vi "Constellation diagram wizard.vi"() -> ()   [LabVIEW 2010]
uses:
  <vilib>/Waveform/DTblOps.llb/DTbl Invert Digital.vi
  <vilib>/Waveform/DTblOps.llb/DTbl Digital Size.vi
  <vilib>/Waveform/DTblOps.llb/DTbl Digital to Binary U32.vi
panel:
  in  "Цвет подписей точек":u32(colorbox)=6618880
  in  "Перемешать соотношения":bool
  out "digital waveform":digitalwaveform(waveform)={"t0"=timestamp(0 s since 1904-01-01), "dt"=0.01, "Y"={"transitions"=[], "data"=[[1, 0, 0], [0, 0, 1], [1, 0, 1], [0, 1, 1], [0, 0, 0], [1, 0, 0], [0, 0, 1], [0, 0, 0], [1, 1, 0], [1, 0, 0], [0, 1, 0], [0, 1, 0], [0, 1, 0], [0, 1, 1], [0, 1, 1], [1, 1, 1], [1, 0, 1], [0, 1, 0], [1, 0, 1], [1, 0, 1], [0, 0, 1], [0, 1, 0], [0, 1, 1], [1, 0, 1], [1, 0, 0], [1, 1, 0], [1, 1, 1], [1, 0, 0], [1, 0, 1], [1, 0, 1], [0, 1, 0], [0, 1, 1], [1, 1, 1], [0, 1, 0], [1, 1, 0], [1, 0, 0], [1, 0, 0], [0, 0, 0], [1, 0, 1], [0, 1, 1], [0, 1, 1], [0, 0, 0], [1, 1, 1], [0, 0, 1], [0, 1, 1], [0, 0, 0], [0, 1, 1], [0, 1, 0], [1, 1, 1], [1, 1, 1], [1, 0, 0], [1, 1, 1], [1, 0, 0], [0, 1, 1], [1, 0, 1], [0, 1, 0], [1, 0, 0], [0, 0, 1], [1, 0, 0], [0, 1, 0], [0, 0, 0], [1, 0, 1], [1, 0, 0], [0, 1, 1], [0, 0, 1], [1, 1, 0], [0, 0, 1], [1, 0, 1], [0, 0, 1], [0, 0, 1], [1, 1, 1], [0, 1, 0], [1, 1, 0], [0, 0, 1], [0, 0, 0], [1, 1, 1], [0, 1, 1], [0, 0, 0], [0, 0, 0], [0, 0, 1], [0, 0, 1], [1, 0, 0], [0, 1, 1], [0, 1, 1], [1, 1, 0], [1, 0, 0], [1, 1, 0], [0, 0, 1], [1, 1, 0], [1, 1, 1], [0, 0, 1], [0, 0, 1], [1, 1, 0], [1, 0, 1], [0, 0, 0], [1, 1, 0], [0, 0, 0], [0, 0, 1], [1, 1, 0], [0, 1, 0]]}}
  out "Количество ПБ":ext=8.0
  out "Временная диаграмма каналов":digitalwaveform(graph)={"t0"=timestamp(0 s since 1904-01-01), "dt"=0.01, "Y"={"transitions"=[], "data"=[[1, 0, 0], [0, 0, 1], [1, 0, 1], [0, 1, 1], [0, 0, 0], [1, 0, 0], [0, 0, 1], [0, 0, 0], [1, 1, 0], [1, 0, 0], [0, 1, 0], [0, 1, 0], [0, 1, 0], [0, 1, 1], [0, 1, 1], [1, 1, 1], [1, 0, 1], [0, 1, 0], [1, 0, 1], [1, 0, 1], [0, 0, 1], [0, 1, 0], [0, 1, 1], [1, 0, 1], [1, 0, 0], [1, 1, 0], [1, 1, 1], [1, 0, 0], [1, 0, 1], [1, 0, 1], [0, 1, 0], [0, 1, 1], [1, 1, 1], [0, 1, 0], [1, 1, 0], [1, 0, 0], [1, 0, 0], [0, 0, 0], [1, 0, 1], [0, 1, 1], [0, 1, 1], [0, 0, 0], [1, 1, 1], [0, 0, 1], [0, 1, 1], [0, 0, 0], [0, 1, 1], [0, 1, 0], [1, 1, 1], [1, 1, 1], [1, 0, 0], [1, 1, 1], [1, 0, 0], [0, 1, 1], [1, 0, 1], [0, 1, 0], [1, 0, 0], [0, 0, 1], [1, 0, 0], [0, 1, 0], [0, 0, 0], [1, 0, 1], [1, 0, 0], [0, 1, 1], [0, 0, 1], [1, 1, 0], [0, 0, 1], [1, 0, 1], [0, 0, 1], [0, 0, 1], [1, 1, 1], [0, 1, 0], [1, 1, 0], [0, 0, 1], [0, 0, 0], [1, 1, 1], [0, 1, 1], [0, 0, 0], [0, 0, 0], [0, 0, 1], [0, 0, 1], [1, 0, 0], [0, 1, 1], [0, 1, 1], [1, 1, 0], [1, 0, 0], [1, 1, 0], [0, 0, 1], [1, 1, 0], [1, 1, 1], [0, 0, 1], [0, 0, 1], [1, 1, 0], [1, 0, 1], [0, 0, 0], [1, 1, 0], [0, 0, 0], [0, 0, 1], [1, 1, 0], [0, 1, 0]]}}
  out "Точки карты после разметки":cluster{"I":dbl, "Q":dbl, "ПБ":u32}[](array[cluster])=[{"I"=6.0, "Q"=0.0, "ПБ"=4}, {"I"=-4.0, "Q"=4.0, "ПБ"=1}, {"I"=-4.0, "Q"=-4.0, "ПБ"=5}, {"I"=-6.0, "Q"=0.0, "ПБ"=3}, {"I"=0.0, "Q"=6.0, "ПБ"=0}, {"I"=6.0, "Q"=0.0, "ПБ"=4}, {"I"=-4.0, "Q"=4.0, "ПБ"=1}, {"I"=0.0, "Q"=6.0, "ПБ"=0}, {"I"=4.0, "Q"=-4.0, "ПБ"=6}, {"I"=6.0, "Q"=0.0, "ПБ"=4}, {"I"=4.0, "Q"=4.0, "ПБ"=2}, {"I"=4.0, "Q"=4.0, "ПБ"=2}, {"I"=4.0, "Q"=4.0, "ПБ"=2}, {"I"=-6.0, "Q"=0.0, "ПБ"=3}, {"I"=-6.0, "Q"=0.0, "ПБ"=3}, {"I"=0.0, "Q"=-6.0, "ПБ"=7}, {"I"=-4.0, "Q"=-4.0, "ПБ"=5}, {"I"=4.0, "Q"=4.0, "ПБ"=2}, {"I"=-4.0, "Q"=-4.0, "ПБ"=5}, {"I"=-4.0, "Q"=-4.0, "ПБ"=5}, {"I"=-4.0, "Q"=4.0, "ПБ"=1}, {"I"=4.0, "Q"=4.0, "ПБ"=2}, {"I"=-6.0, "Q"=0.0, "ПБ"=3}, {"I"=-4.0, "Q"=-4.0, "ПБ"=5}, {"I"=6.0, "Q"=0.0, "ПБ"=4}, {"I"=4.0, "Q"=-4.0, "ПБ"=6}, {"I"=0.0, "Q"=-6.0, "ПБ"=7}, {"I"=6.0, "Q"=0.0, "ПБ"=4}, {"I"=-4.0, "Q"=-4.0, "ПБ"=5}, {"I"=-4.0, "Q"=-4.0, "ПБ"=5}, {"I"=4.0, "Q"=4.0, "ПБ"=2}, {"I"=-6.0, "Q"=0.0, "ПБ"=3}, {"I"=0.0, "Q"=-6.0, "ПБ"=7}, {"I"=4.0, "Q"=4.0, "ПБ"=2}, {"I"=4.0, "Q"=-4.0, "ПБ"=6}, {"I"=6.0, "Q"=0.0, "ПБ"=4}, {"I"=6.0, "Q"=0.0, "ПБ"=4}, {"I"=0.0, "Q"=6.0, "ПБ"=0}, {"I"=-4.0, "Q"=-4.0, "ПБ"=5}, {"I"=-6.0, "Q"=0.0, "ПБ"=3}, {"I"=-6.0, "Q"=0.0, "ПБ"=3}, {"I"=0.0, "Q"=6.0, "ПБ"=0}, {"I"=0.0, "Q"=-6.0, "ПБ"=7}, {"I"=-4.0, "Q"=4.0, "ПБ"=1}, {"I"=-6.0, "Q"=0.0, "ПБ"=3}, {"I"=0.0, "Q"=6.0, "ПБ"=0}, {"I"=-6.0, "Q"=0.0, "ПБ"=3}, {"I"=4.0, "Q"=4.0, "ПБ"=2}, {"I"=0.0, "Q"=-6.0, "ПБ"=7}, {"I"=0.0, "Q"=-6.0, "ПБ"=7}, {"I"=6.0, "Q"=0.0, "ПБ"=4}, {"I"=0.0, "Q"=-6.0, "ПБ"=7}, {"I"=6.0, "Q"=0.0, "ПБ"=4}, {"I"=-6.0, "Q"=0.0, "ПБ"=3}, {"I"=-4.0, "Q"=-4.0, "ПБ"=5}, {"I"=4.0, "Q"=4.0, "ПБ"=2}, {"I"=6.0, "Q"=0.0, "ПБ"=4}, {"I"=-4.0, "Q"=4.0, "ПБ"=1}, {"I"=6.0, "Q"=0.0, "ПБ"=4}, {"I"=4.0, "Q"=4.0, "ПБ"=2}, {"I"=0.0, "Q"=6.0, "ПБ"=0}, {"I"=-4.0, "Q"=-4.0, "ПБ"=5}, {"I"=6.0, "Q"=0.0, "ПБ"=4}, {"I"=-6.0, "Q"=0.0, "ПБ"=3}, {"I"=-4.0, "Q"=4.0, "ПБ"=1}, {"I"=4.0, "Q"=-4.0, "ПБ"=6}, {"I"=-4.0, "Q"=4.0, "ПБ"=1}, {"I"=-4.0, "Q"=-4.0, "ПБ"=5}, {"I"=-4.0, "Q"=4.0, "ПБ"=1}, {"I"=-4.0, "Q"=4.0, "ПБ"=1}, {"I"=0.0, "Q"=-6.0, "ПБ"=7}, {"I"=4.0, "Q"=4.0, "ПБ"=2}, {"I"=4.0, "Q"=-4.0, "ПБ"=6}, {"I"=-4.0, "Q"=4.0, "ПБ"=1}, {"I"=0.0, "Q"=6.0, "ПБ"=0}, {"I"=0.0, "Q"=-6.0, "ПБ"=7}, {"I"=-6.0, "Q"=0.0, "ПБ"=3}, {"I"=0.0, "Q"=6.0, "ПБ"=0}, {"I"=0.0, "Q"=6.0, "ПБ"=0}, {"I"=-4.0, "Q"=4.0, "ПБ"=1}, {"I"=-4.0, "Q"=4.0, "ПБ"=1}, {"I"=6.0, "Q"=0.0, "ПБ"=4}, {"I"=-6.0, "Q"=0.0, "ПБ"=3}, {"I"=-6.0, "Q"=0.0, "ПБ"=3}, {"I"=4.0, "Q"=-4.0, "ПБ"=6}, {"I"=6.0, "Q"=0.0, "ПБ"=4}, {"I"=4.0, "Q"=-4.0, "ПБ"=6}, {"I"=-4.0, "Q"=4.0, "ПБ"=1}, {"I"=4.0, "Q"=-4.0, "ПБ"=6}, {"I"=0.0, "Q"=-6.0, "ПБ"=7}, {"I"=-4.0, "Q"=4.0, "ПБ"=1}, {"I"=-4.0, "Q"=4.0, "ПБ"=1}, {"I"=4.0, "Q"=-4.0, "ПБ"=6}, {"I"=-4.0, "Q"=-4.0, "ПБ"=5}, {"I"=0.0, "Q"=6.0, "ПБ"=0}, {"I"=4.0, "Q"=-4.0, "ПБ"=6}, {"I"=0.0, "Q"=6.0, "ПБ"=0}, {"I"=-4.0, "Q"=4.0, "ПБ"=1}, {"I"=4.0, "Q"=-4.0, "ПБ"=6}, {"I"=4.0, "Q"=4.0, "ПБ"=2}] {"ПБ" items=["0", "1", "10", "11", "100", "101", "110", "111"]}
  in  "Все возможные точки карты":cluster{"I":dbl, "Q":dbl, "ПБ":u32}[](array[cluster])=[{"I"=0.0, "Q"=6.0, "ПБ"=0}, {"I"=-4.0, "Q"=4.0, "ПБ"=1}, {"I"=4.0, "Q"=4.0, "ПБ"=2}, {"I"=-6.0, "Q"=0.0, "ПБ"=3}, {"I"=6.0, "Q"=0.0, "ПБ"=4}, {"I"=-4.0, "Q"=-4.0, "ПБ"=5}, {"I"=4.0, "Q"=-4.0, "ПБ"=6}, {"I"=0.0, "Q"=-6.0, "ПБ"=7}] {"ПБ" items=["0", "1", "10", "11", "100", "101", "110", "111"]}
  in  "Соотношение точек с ПБ":u8(ring) items=["По возрастанию", "По убыванию", "Пользовательское"]
  in  "Стоп":bool
  in  "Интервалы и смещения":T1={"Q смещение"=0.0, "Q интервал"=2.0, "I смещение"=0.0, "I интервал"=2.0} {"I интервал" min=1.0 step=1.0; "Q интервал" min=1.0 step=1.0}
  out "Количество точек":i32=8
  in  "Добавлять точки при\nувеличении размера карты":bool=TRUE
  in  "Очистить полностью":bool
  in  "Заполнить полностью":bool
  in  "Точки карты (позиции)":bool[][](array[boolean])=[[FALSE, FALSE, FALSE, TRUE, FALSE, FALSE, FALSE], [FALSE, TRUE, FALSE, FALSE, FALSE, TRUE, FALSE], [FALSE, FALSE, FALSE, FALSE, FALSE, FALSE, FALSE], [TRUE, FALSE, FALSE, FALSE, FALSE, FALSE, TRUE], [FALSE, FALSE, FALSE, FALSE, FALSE, FALSE, FALSE], [FALSE, TRUE, FALSE, FALSE, FALSE, TRUE, FALSE], [FALSE, FALSE, FALSE, TRUE, FALSE, FALSE, FALSE]]
  in  "Размер карты (N*N)":i32(slide)=7 min=1 max=8 step=1 scale=0.0..8.0
  in  "Показать подписи точек на карте":bool=TRUE
  in  "Смещение подписей":cluster{"I":dbl, "Q":dbl}={"I"=0.0, "Q"=0.5}
  in  "Путь для загрузки карты":path=path "C:/Users/fl1ckje/Desktop/OFDM/map.xml"
  in  "Загрузить карту из файла":bool
  in  "Путь для сохранения карты":path=path "C:/Users/fl1ckje/Desktop/OFDM/map.xml"
  in  "Сохранить карту в файл":bool
  out "Карта":cluster{cluster{"I":dbl, "Q":dbl}[]}[](graph)=[{[{"I"=0.0, "Q"=6.0}, {"I"=-4.0, "Q"=4.0}, {"I"=4.0, "Q"=4.0}, {"I"=-6.0, "Q"=0.0}, {"I"=6.0, "Q"=0.0}, {"I"=-4.0, "Q"=-4.0}, {"I"=4.0, "Q"=-4.0}, {"I"=0.0, "Q"=-6.0}]}, {[{"I"=10.0, "Q"=0.0}, {"I"=-10.0, "Q"=0.0}, {"I"=0.0, "Q"=10.0}, {"I"=0.0, "Q"=-10.0}]}]
  out "Карта 2":cluster{cluster{"I":dbl, "Q":dbl}[]}[](graph)=[{[{"I"=4.0, "Q"=4.0}, {"I"=0.0, "Q"=-6.0}, {"I"=6.0, "Q"=0.0}, {"I"=-6.0, "Q"=0.0}, {"I"=0.0, "Q"=-6.0}, {"I"=0.0, "Q"=-6.0}, {"I"=0.0, "Q"=-6.0}, {"I"=-4.0, "Q"=4.0}, {"I"=0.0, "Q"=-6.0}, {"I"=4.0, "Q"=4.0}, {"I"=4.0, "Q"=4.0}, {"I"=0.0, "Q"=6.0}, {"I"=-6.0, "Q"=0.0}, {"I"=-4.0, "Q"=-4.0}, {"I"=-4.0, "Q"=4.0}, {"I"=-4.0, "Q"=4.0}, {"I"=-6.0, "Q"=0.0}, {"I"=-4.0, "Q"=4.0}, {"I"=0.0, "Q"=6.0}, {"I"=-4.0, "Q"=4.0}, {"I"=-4.0, "Q"=4.0}, {"I"=0.0, "Q"=-6.0}, {"I"=-4.0, "Q"=-4.0}, {"I"=6.0, "Q"=0.0}, {"I"=-6.0, "Q"=0.0}, {"I"=-4.0, "Q"=-4.0}, {"I"=0.0, "Q"=-6.0}, {"I"=4.0, "Q"=4.0}, {"I"=-4.0, "Q"=4.0}, {"I"=4.0, "Q"=-4.0}, {"I"=-4.0, "Q"=-4.0}, {"I"=-4.0, "Q"=-4.0}, {"I"=0.0, "Q"=-6.0}, {"I"=-6.0, "Q"=0.0}, {"I"=0.0, "Q"=-6.0}, {"I"=6.0, "Q"=0.0}, {"I"=0.0, "Q"=-6.0}, {"I"=-4.0, "Q"=4.0}, {"I"=4.0, "Q"=-4.0}, {"I"=6.0, "Q"=0.0}, {"I"=4.0, "Q"=4.0}, {"I"=6.0, "Q"=0.0}, {"I"=4.0, "Q"=4.0}, {"I"=0.0, "Q"=-6.0}, {"I"=-4.0, "Q"=4.0}, {"I"=6.0, "Q"=0.0}, {"I"=-4.0, "Q"=4.0}, {"I"=-4.0, "Q"=4.0}, {"I"=4.0, "Q"=4.0}, {"I"=6.0, "Q"=0.0}, {"I"=-4.0, "Q"=4.0}, {"I"=4.0, "Q"=4.0}, {"I"=0.0, "Q"=-6.0}, {"I"=0.0, "Q"=6.0}, {"I"=-4.0, "Q"=4.0}, {"I"=-6.0, "Q"=0.0}, {"I"=6.0, "Q"=0.0}, {"I"=-4.0, "Q"=4.0}, {"I"=-4.0, "Q"=4.0}, {"I"=0.0, "Q"=-6.0}, {"I"=6.0, "Q"=0.0}, {"I"=0.0, "Q"=-6.0}, {"I"=-4.0, "Q"=-4.0}, {"I"=0.0, "Q"=-6.0}, {"I"=-6.0, "Q"=0.0}, {"I"=4.0, "Q"=4.0}, {"I"=4.0, "Q"=4.0}, {"I"=4.0, "Q"=4.0}, {"I"=0.0, "Q"=-6.0}, {"I"=-4.0, "Q"=-4.0}, {"I"=0.0, "Q"=-6.0}, {"I"=0.0, "Q"=-6.0}, {"I"=0.0, "Q"=-6.0}, {"I"=0.0, "Q"=-6.0}, {"I"=-6.0, "Q"=0.0}, {"I"=4.0, "Q"=4.0}, {"I"=-4.0, "Q"=-4.0}, {"I"=4.0, "Q"=-4.0}, {"I"=-6.0, "Q"=0.0}, {"I"=4.0, "Q"=4.0}, {"I"=0.0, "Q"=6.0}, {"I"=4.0, "Q"=4.0}, {"I"=-6.0, "Q"=0.0}, {"I"=4.0, "Q"=-4.0}, {"I"=0.0, "Q"=-6.0}, {"I"=0.0, "Q"=6.0}, {"I"=4.0, "Q"=-4.0}, {"I"=0.0, "Q"=-6.0}, {"I"=4.0, "Q"=-4.0}, {"I"=-4.0, "Q"=4.0}, {"I"=6.0, "Q"=0.0}, {"I"=-4.0, "Q"=4.0}, {"I"=-4.0, "Q"=4.0}, {"I"=4.0, "Q"=-4.0}, {"I"=0.0, "Q"=6.0}, {"I"=4.0, "Q"=-4.0}, {"I"=6.0, "Q"=0.0}, {"I"=4.0, "Q"=4.0}, {"I"=0.0, "Q"=6.0}, {"I"=-4.0, "Q"=4.0}]}, {[{"I"=10.0, "Q"=0.0}, {"I"=-10.0, "Q"=0.0}, {"I"=0.0, "Q"=10.0}, {"I"=0.0, "Q"=-10.0}]}] caption="Карта"
  in  "Воспроизвести":bool
  in  "Источник БП":u16(ring) items=["Случайный", "Wav файл"]
  in  "Построить карту с помощью разметки":bool
  in  "глубина кодирования (бит)":i32=8
  in  "Путь к wav файлу":path=path "C:/Users/fl1ckje/Desktop/OFDM/test.wav"
  in  "Частота дискретизации случайной последовательности":dbl=100.0 min=100.0 max=200000.0 format="%#_13f"
  in  "Количество каналов":i32=3 min=1 max=6 step=1
  # "Редактор разметки карты"
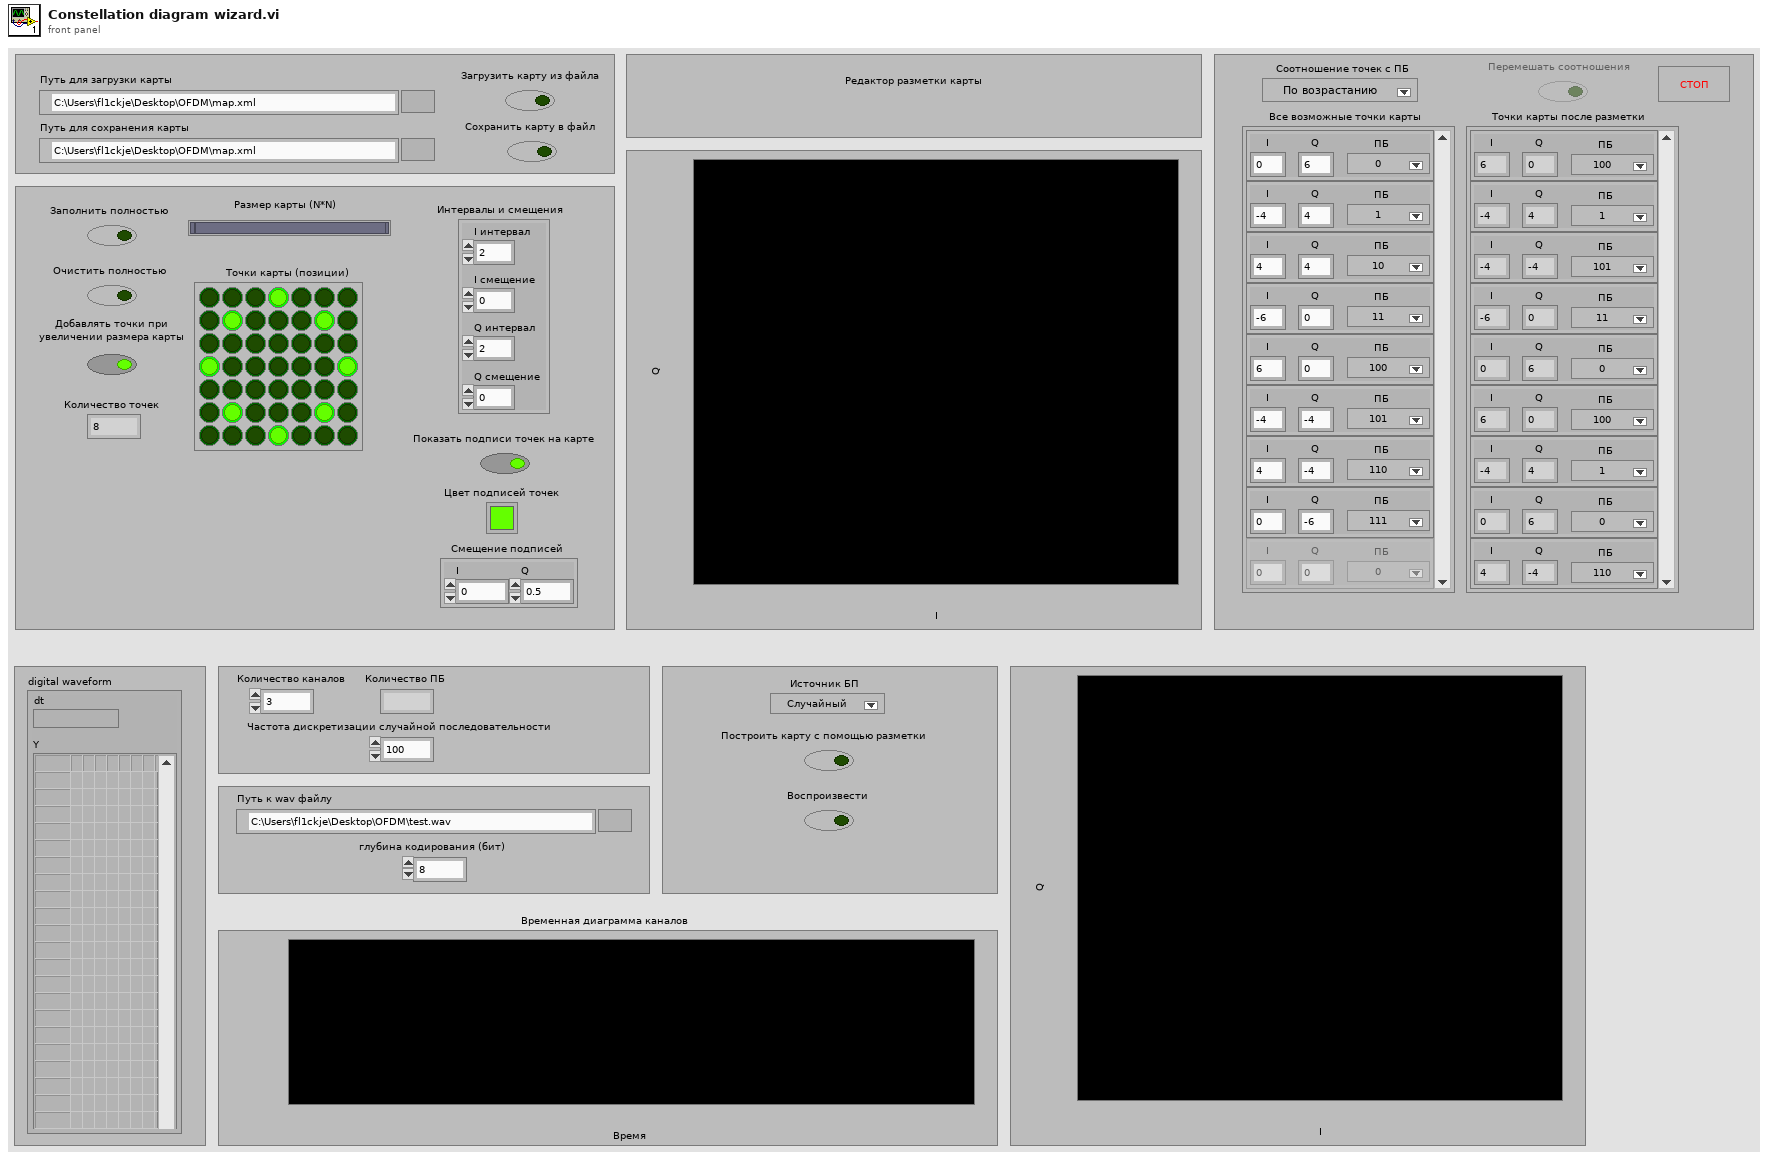
[diagram p1: front panel]
types:
  T1 = cluster{"Q смещение":dbl, "Q интервал":dbl, "I смещение":dbl, "I интервал":dbl}
  T2 = cluster{i16[][], "Value":cluster{"Q смещение":dbl, "Q интервал":dbl, "I смещение":dbl, "I интервал":dbl}, "Value":cluster{"I":dbl, "Q":dbl, "Биты":u32}[], "Value":u8}
  T3 = enum8{"Enabled", "Disabled", "Disabled and Grayed Out"}
  T4 = enum16{"open", "open or create", "create or replace", "create", "open (read only)"}
  T5 = cluster{"Name":string, "Color":u32, "Style":u8, "Point Style":u8, "Name Visible":bool, "Allow Drag":bool, "Annotation Mode":u32, "Plot":i32, "Index":i32, "Position":cluster{"X":dbl, "Y":dbl}, "X Scale":u32, "Y Scale":u32, "Show Arrow":bool, "Lock Name":bool, "Plot Area":i32, "Label Offset":cluster{"X":dbl, "Y":dbl}}
  T6 = cluster{"Name":string, "Color":u32, "Style":u8, "Point Style":u8, "Name Visible":bool, "Allow Drag":bool, "Annotation Mode":u32, "Plot":i32, "Index":i32, "Position":cluster{"X":dbl, "Y":dbl}, "X Scale":u32, "Y Scale":u32, "Show Arrow":bool, "Lock Name":bool, "Plot Area":i32, "Label Offset":cluster{"X":dbl, "Y":dbl}}[]
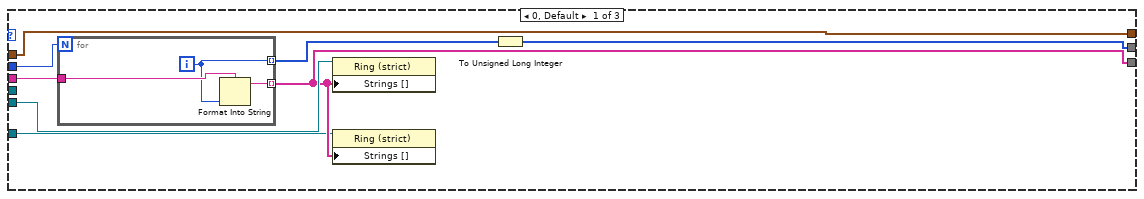
[diagram p2: hidden frame]
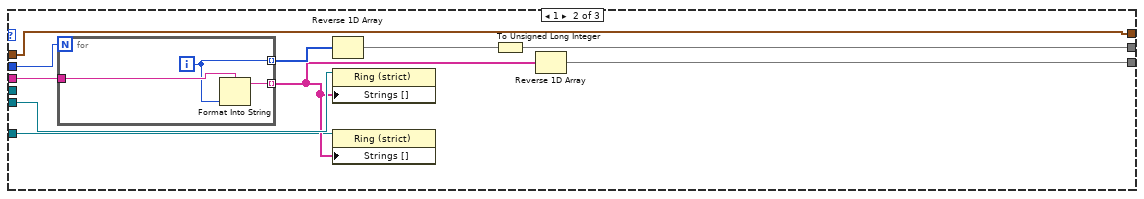
[diagram p3: hidden frame]
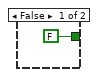
[diagram p4: hidden frame]
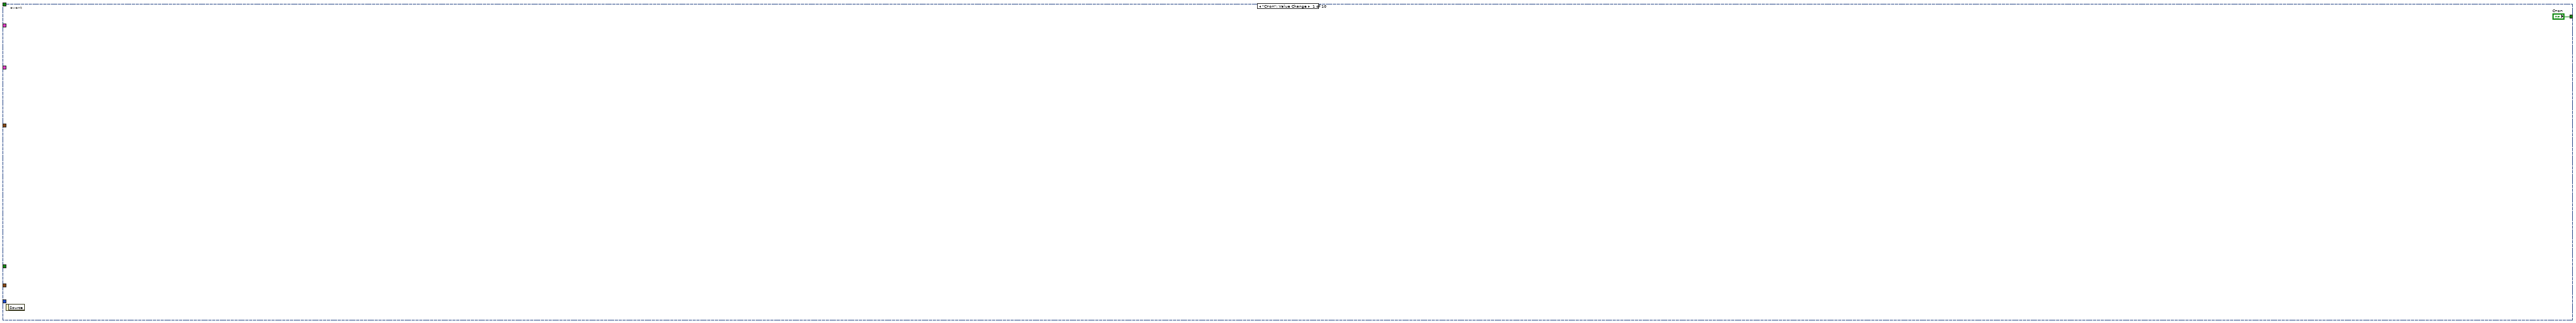
[diagram p6: hidden frame]
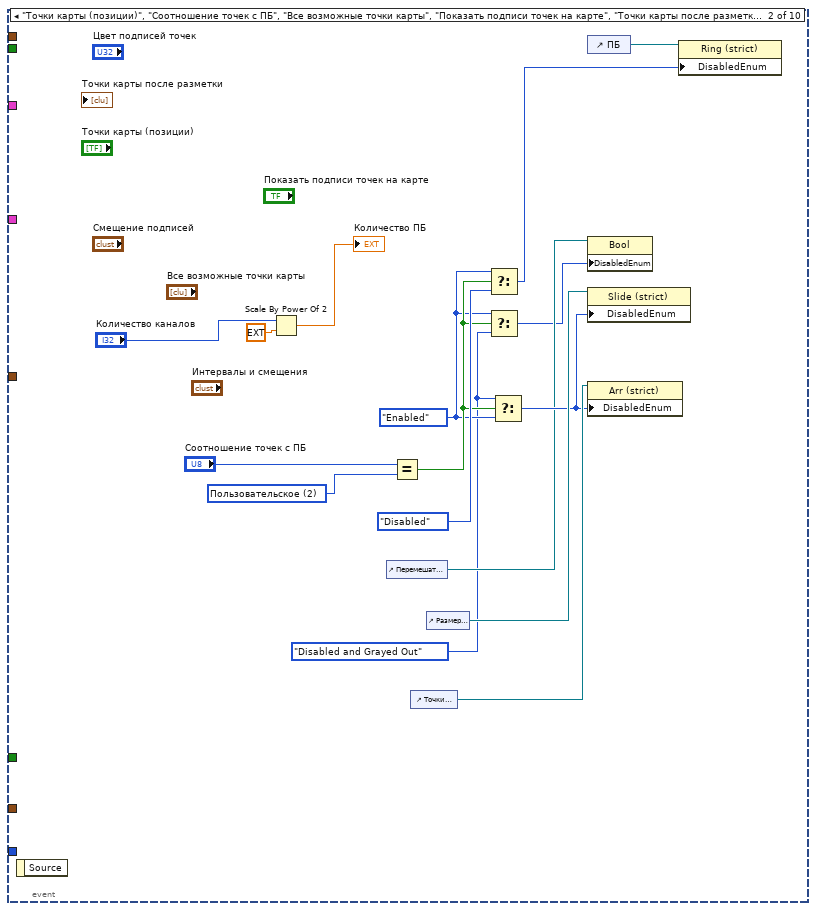
[diagram p7: hidden frame]
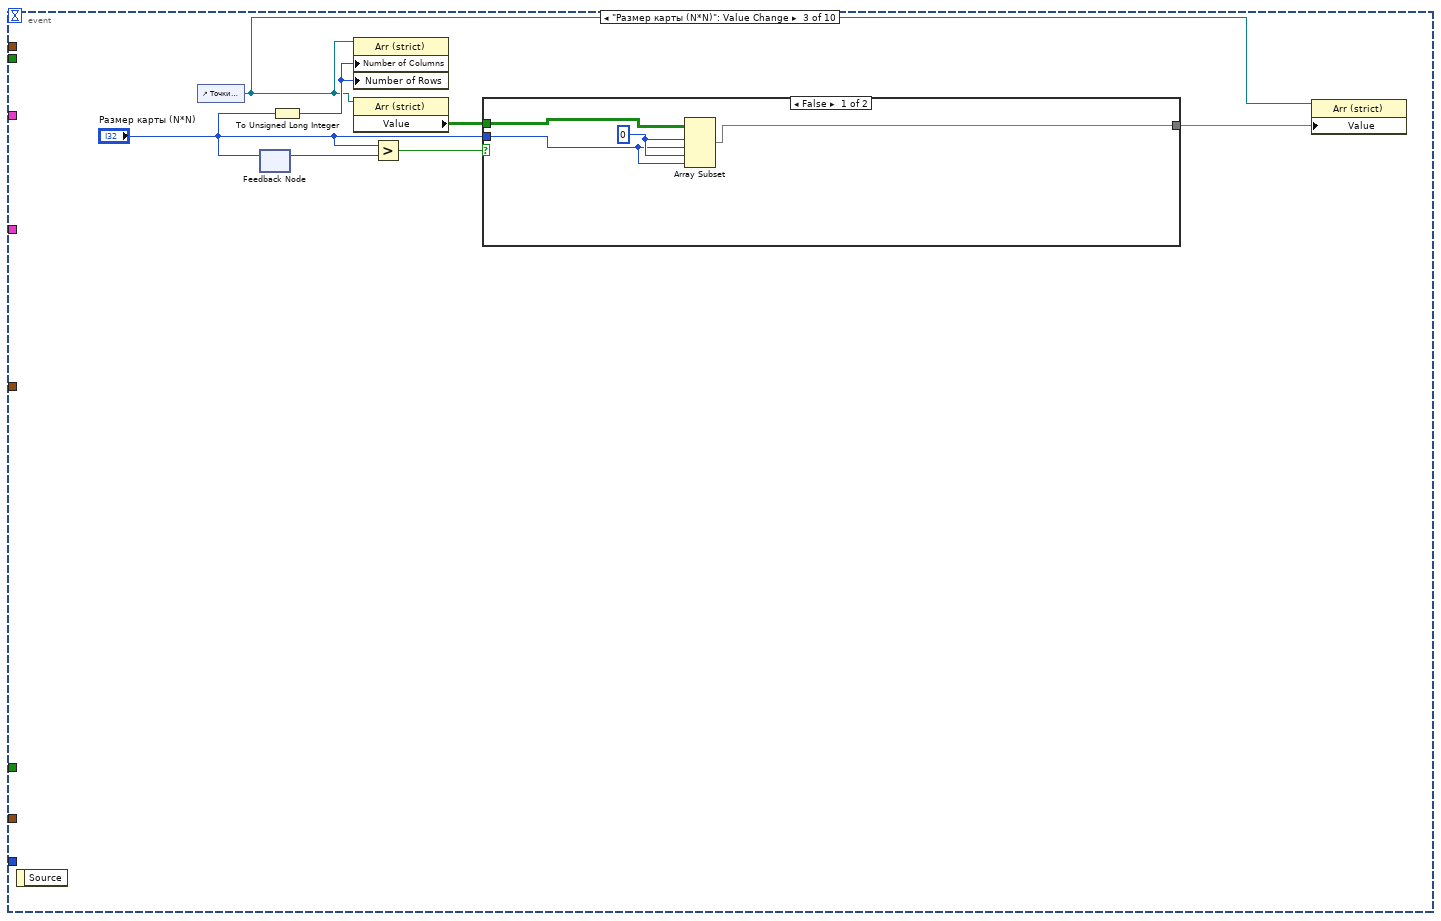
[diagram p8: hidden frame]
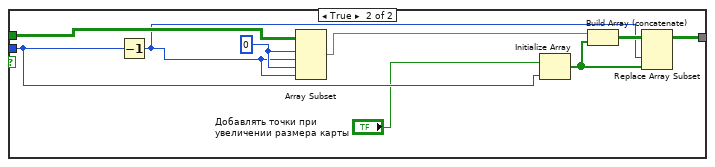
[diagram p9: hidden frame]
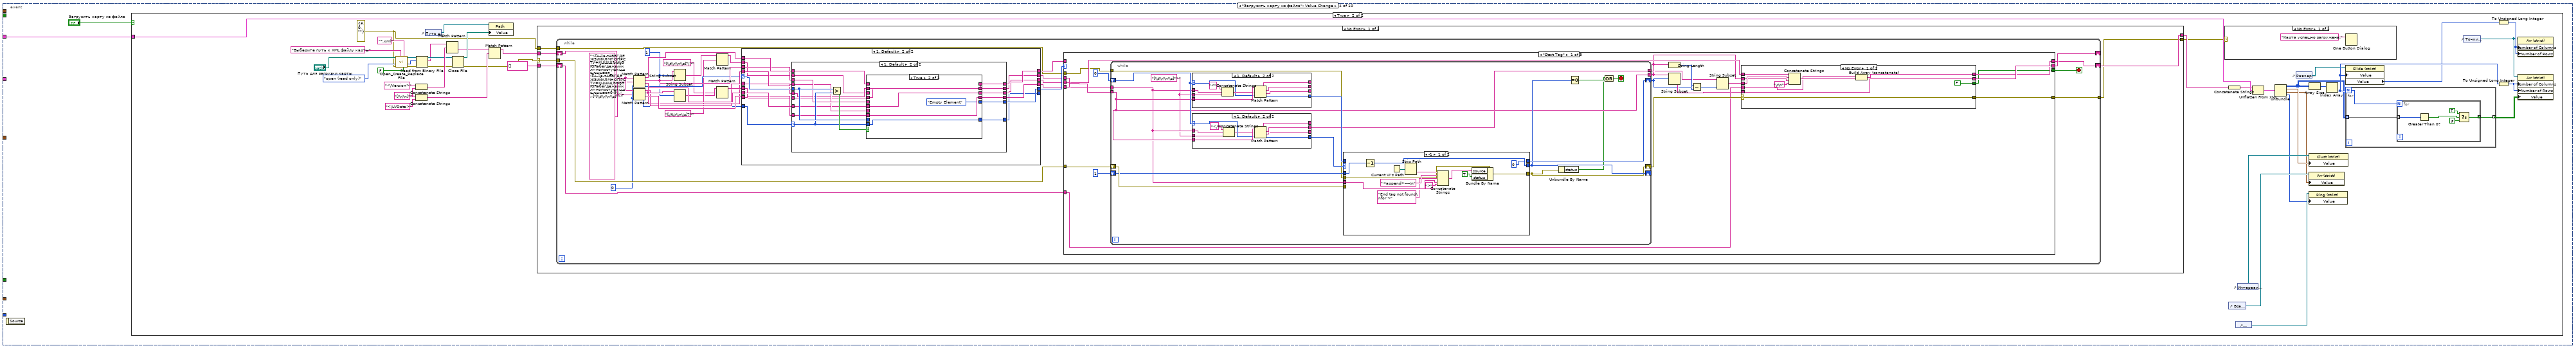
[diagram p10: hidden frame]
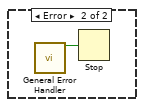
[diagram p12: hidden frame]
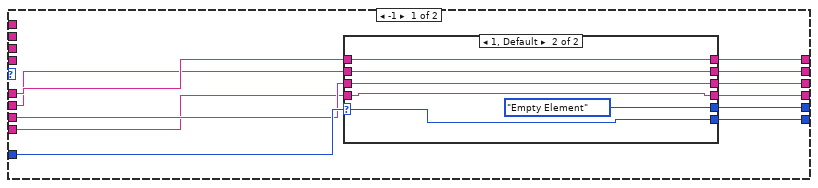
[diagram p13: hidden frame]
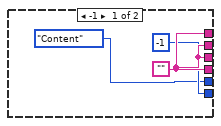
[diagram p14: hidden frame]
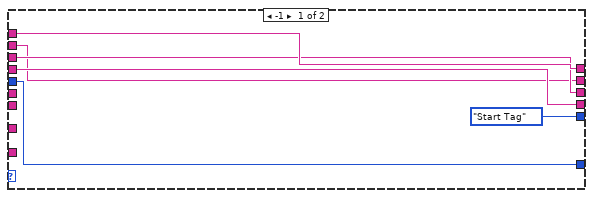
[diagram p15: hidden frame]
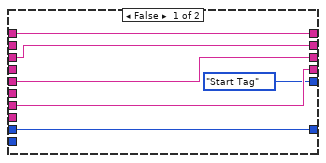
[diagram p16: hidden frame]
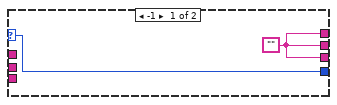
[diagram p17: hidden frame]
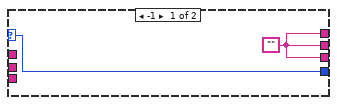
[diagram p18: hidden frame]
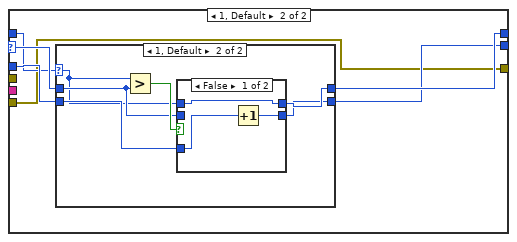
[diagram p19: hidden frame]
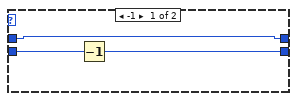
[diagram p20: hidden frame]
diagram:
  n1 = while {
    stop <- w63 stop-if-true
    w14 = TRUE ("Lock Name")
    w15 = T5 {"Name"="", "Color"=0, "Style"=0, "Point Style"=0, "Name Visible"=FALSE, "Allow Drag"=FALSE, "Annotation Mode"=0, "Plot"=0, "Index"=0, "Position"={"X"=0.0, "Y"=0.0}, "X Scale"=0, "Y Scale"=0, "Show Arrow"=FALSE, "Lock Name"=FALSE, "Plot Area"=0, "Label Offset"={"X"=0.0, "Y"=0.0}} ("Cluster")
    w38 = -0.5 ("y")
    w55 = 0.0 ("Q")
    w17 = cluster{"I":dbl, "Q":dbl} {"I"=0.0, "Q"=0.0}  # I, Q
    n2 = control-ref of="Интервалы и смещения"() -> (w32:refnum<vi>)
    n3 = control-ref of="Размер карты (N*N)"() -> (w60:refnum<vi>)
    n4 = property class="Clust (strict)"(reference=w32) -> ("Value"=w31:T1)  [unwired: 1 in, 2 out]
    n5 = property class="Slide (strict)"(reference=w60) -> ("Value"=w59:i32)  [unwired: 1 in, 2 out]
    n6 = Unbundle By Name(w31) -> ("I смещение"=w27:dbl, "I интервал"=w28:dbl, "Q интервал"=w30:dbl, "Q смещение"=w29:dbl)
    n7 = Multiply(x=w28, y=w38) -> (x*y=w48:dbl)
    n8 = Multiply(x=w38, y=w30) -> (x*y=w45:dbl)
    n9 = To Double Precision Float(number=w59) -> (double precision float=w47:dbl)
    n10 = Negate(x=w48) -> (-x=w49:dbl)
    n11 = Multiply(x=w47, y=w48) -> (x*y=w52:dbl)
    n12 = Negate(x=w45) -> (-x=w44:dbl)
    n13 = Multiply(x=w47, y=w45) -> (x*y=w46:dbl)
    n14 = Add(x=w52, y=w49) -> (x+y=w50:dbl)
    n15 = Add(x=w46, y=w44) -> (x+y=w43:dbl)
    n16 = Add(x=w27, y=w50) -> (x+y=w40:dbl)
    n17 = Add(x=w43, y=w29) -> (x+y=w51:dbl)
    n18 = for {
      N: w59 -> [_]
      tunnel: [w150] -> w42 mode=indexing
      tunnel: w30 -> [w144]
      tunnel: w51 -> [w142]
      tunnel: w28 -> [w149]
      tunnel: w40 -> [w147]
      tunnel: [w146] -> w39 mode=indexing
      i -> [w151]
      n19 = To Double Precision Float(number=w151) -> (double precision float=w145:dbl)
      n20 = Multiply(x=w149, y=w145) -> (x*y=w148:dbl)
      n21 = Multiply(x=w145, y=w144) -> (x*y=w143:dbl)
      n22 = Add(x=w147, y=w148) -> (x+y=w146:dbl)
      n23 = Add(x=w143, y=w142) -> (x+y=w150:dbl)
    }
    n24 = for {
      tunnel: w42 -> [w156]
      tunnel: [w154] -> w67 mode=indexing
      tunnel: w39 -> [w152] mode=indexing
      tunnel: w17 -> [w153]
      n25 = for {
        tunnel: w152 -> [w160]
        tunnel: w156 -> [w157] mode=indexing
        tunnel: [w159] -> w155 mode=indexing
        tunnel: w153 -> [w158]
        n26 = Bundle By Name(cluster=w158, "I"=w160, "Q"=w157) -> (w159:cluster{"I":dbl, "Q":dbl})
      }
      n27 = Reverse 1D Array(array=w155) -> (reversed array=w154:cluster{"I":dbl, "Q":dbl}[])
    }
    n28 = control-ref of="Точки карты (позиции)"() -> (w62:refnum<vi>)
    n29 = property class="Arr (strict)"(reference=w62) -> ("Value"=w61:bool[][])  [unwired: 1 in, 2 out]
    n30 = Transpose 2D Array(2D array=w67) -> (transposed array=w66:cluster{"I":dbl, "Q":dbl}[][])
    n31 = Square(x=w59) -> (x^2=w37:i32)
    n32 = Reshape Array(w66, w37) -> (w65:cluster{"I":dbl, "Q":dbl}[])
    n33 = Reshape Array(w61, w37) -> (w64:bool[])
    n34 = control-ref of="Соотношение точек с ПБ"() -> (w26:refnum<vi>)
    n35 = for {
      tunnel: w65 -> [w137] mode=indexing
      tunnel: w64 -> [w136] mode=indexing
      shift-right: [w134] -> w22
      shift-left: cluster{"I":dbl, "Q":dbl}[] [] ("Array") -> [w135]
      n36 = case shown="True" w136 {
        tunnel: w135 -> [w138 w140]
        tunnel: w137 -> [_ w139]
        tunnel: [w138 w141] -> w134
        frame False {
        }
        frame True {
          n37 = Build Array (concatenate)(w140, w139) -> (w141:cluster{"I":dbl, "Q":dbl}[])
        }
      }
    }
    n38 = control-ref of="Все возможные точки карты"() -> (w36:refnum<vi>)
    n39 = property class="Ring (strict)"(reference=w26) -> ("Value"=w25:u8)  [unwired: 1 in, 2 out]
    n40 = Array Size(array=w22) -> (size(s)=w24:i32)
    "Количество точек" <- w24
    n41 = control-ref of="ПБ"() -> (w20:refnum<vi>)
    n42 = control-ref of="ПБ"() -> (w6:refnum<vi>)
    n43 = case shown="2" w25 {
      tunnel: w36 -> [_ _ w98]
      tunnel: w24 -> [w74 w86 w96]
      tunnel: [w70 w81 w93] -> w2
      tunnel: "%b" ("format string") -> [w75 w88 w92]
      tunnel: [w73 w85 w97] -> w18
      tunnel: w22 -> [w73 w85 w97]
      tunnel: [w69 w84 w94] -> w21
      tunnel: w20 -> [w72 w83 _]
      tunnel: w6 -> [w68 w79 _]
      frame 0, Default {
        n44 = for {
          N: w74 -> [_]
          tunnel: w75 -> [w78]
          tunnel: [w77] -> w71 mode=indexing
          tunnel: [w76] -> w69 mode=indexing
          i -> [w77]
          n45 = Format Into String(format string=w78, w77) -> (resulting string=w76:string)  [unwired: 2 in, 1 out]
        }
        n46 = property class="Ring (strict)"(reference=w72, "Strings []"=w69) -> ()  [unwired: 1 in, 2 out]
        n47 = property class="Ring (strict)"(reference=w68, "Strings []"=w69) -> ()  [unwired: 1 in, 2 out]
        n48 = To Unsigned Long Integer(number=w71) -> (unsigned 32bit integer=w70:u32[])
      }
      frame 1 {
        n49 = for {
          N: w86 -> [_]
          tunnel: w88 -> [w91]
          tunnel: [w89] -> w87 mode=indexing
          tunnel: [w90] -> w80 mode=indexing
          i -> [w89]
          n50 = Format Into String(format string=w91, w89) -> (resulting string=w90:string)  [unwired: 2 in, 1 out]
        }
        n51 = Reverse 1D Array(array=w87) -> (reversed array=w82:i32[])
        n52 = property class="Ring (strict)"(reference=w83, "Strings []"=w80) -> ()  [unwired: 1 in, 2 out]
        n53 = property class="Ring (strict)"(reference=w79, "Strings []"=w80) -> ()  [unwired: 1 in, 2 out]
        n54 = To Unsigned Long Integer(number=w82) -> (unsigned 32bit integer=w81:u32[])
        n55 = Reverse 1D Array(array=w80) -> (reversed array=w84:string[])
      }
      frame 2 {
        n56 = property class="Arr (strict)"(reference=w98) -> ("Value"=w95:cluster{"I":dbl, "Q":dbl, "ПБ":u32}[])  [unwired: 1 in, 2 out]
        n57 = for {
          N: w96 -> [_]
          tunnel: w95 -> [w118] mode=indexing
          tunnel: [w121] -> w93 mode=indexing
          tunnel: [w120] -> w94 mode=indexing
          tunnel: w92 -> [w119]
          n58 = Unbundle By Name(w118) -> ("ПБ"=w121:u32)
          n59 = Format Into String(format string=w119, w121) -> (resulting string=w120:string)  [unwired: 2 in, 1 out]
        }
        n60 = for {
          tunnel: w93 -> [w103] mode=indexing
          tunnel: w93 -> [w101]
          tunnel: w92 -> [w100]
          i -> [w104]
          stop <- w99 stop-if-true
          n61 = Delete From Array(array=w101, index=w104) -> (array with subset deleted=w102:u32[])  [unwired: 1 in, 1 out]
          n62 = for {
            tunnel: w103 -> [w109]
            tunnel: w102 -> [w107] mode=indexing
            tunnel: w100 -> [w106]
            tunnel: [w105] -> w99
            stop <- w105 stop-if-true
            n63 = Equal?(x=w109, y=w107) -> (x = y?=w108:bool)
            n64 = case shown="True" w108 {
              tunnel: w107 -> [_ w117]
              tunnel: w106 -> [_ w116]
              tunnel: [FALSE ("true") w115] -> w105
              frame False {
              }
              frame True {
                n65 = Format Into String(format string=w116, w117) -> (resulting string=w112:string)  [unwired: 2 in, 1 out]
                n66 = Concatenate Strings("Последовательность битов \"" ("message"), w112, "\" повторяется в разметке!") -> (w113:string)
                n67 = One Button Dialog(message=w113) -> (true=w115:bool)  [unwired: 1 in]
              }
            }
          }
        }
      }
    }
    n68 = control-ref of="Показать подписи точек на карте"() -> (w23:refnum<vi>)
    n69 = control-ref of="Смещение подписей"() -> (w19:refnum<vi>)
    n70 = control-ref of="Цвет подписей точек"() -> (w5:refnum<vi>)
    n71 = property class="Clust (strict)"(reference=w19) -> ("Value"=w13:cluster{"X":dbl, "Y":dbl})  [unwired: 1 in, 2 out]
    n72 = property class="Bool (strict)"(reference=w23) -> ("Value"=w12:bool)  [unwired: 1 in, 2 out]
    n73 = property class="ColBox"(reference=w5) -> ("Value"=w4:u32)  [unwired: 1 in, 2 out]
    n74 = for {
      tunnel: w18 -> [w133] mode=indexing
      tunnel: [w132] -> w35 mode=indexing
      tunnel: w2 -> [w131] mode=indexing
      tunnel: w21 -> [w130] mode=indexing
      tunnel: [w129] -> w33 mode=indexing
      tunnel: w13 -> [w128]
      tunnel: w12 -> [w127]
      tunnel: w4 -> [w126]
      tunnel: w15 -> [w125]
      tunnel: w14 -> [w124]
      n75 = Unbundle By Name(w133) -> ("I"=w123:dbl, "Q"=w122:dbl)
      n76 = Bundle By Name(cluster=w125, "Position.X"=w123, "Position.Y"=w122, "Name"=w130, "Lock Name"=w124, "Name Visible"=w127, "Label Offset"=w128, "Color"=w126) -> (w129:T5)
      n77 = Bundle("I"=w123, "Q"=w122, "ПБ"=w131) -> (w132:cluster{"I":dbl, "Q":dbl, "ПБ":u32})  [unwired: 1 in]
    }
    n78 = control-ref of="Карта"() -> (w58:refnum<vi>)
    n79 = property class="Arr (strict)"(reference=w36, "Value"=w35) -> ()  [unwired: 1 in, 2 out]
    n80 = property class="XYGraph (strict)"(reference=w58, "AnntList"=w33) -> ("XScale.Maximum"=w8:dbl, "XScale.Minimum"=w9:dbl, "YScale.Maximum"=w11:dbl, "YScale.Minimum"=w10:dbl)  [unwired: 1 in, 2 out]
    n81 = Bundle By Name(cluster=w17, "I"=w8, "Q"=w55) -> (w57:cluster{"I":dbl, "Q":dbl})
    n82 = Bundle By Name(cluster=w17, "I"=w9, "Q"=w55) -> (w56:cluster{"I":dbl, "Q":dbl})
    n83 = Bundle By Name(cluster=w17, "I"=w55, "Q"=w11) -> (w54:cluster{"I":dbl, "Q":dbl})
    n84 = Bundle By Name(cluster=w17, "I"=w55, "Q"=w10) -> (w53:cluster{"I":dbl, "Q":dbl})
    n85 = Build Array(w57, w56, w54, w53) -> (w16:cluster{"I":dbl, "Q":dbl}[])
    n86 = Build Cluster Array(w18, w16) -> (→"Карта":cluster{"Array":cluster{"I":dbl, "Q":dbl}[]}[])
    n87 = event shown="[4] \"Построить карту с помощью разметки\": Value Change" {
      selector: _ -> [_ _ _ _ _ _ _ _ _ _]
      dyn-events: _ -> [_ _ _ _ _ _ _ _ _ _]
      timeout: -1 -> [_ _ _ _ _ _ _ _ _ _]
      tunnel: ["Стоп" _ _ _ _ _ _ _ _ _] -> w63
      tunnel: w17 -> [_ _ _ _ w486 _ _ _ _ _]
      tunnel: w16 -> [_ _ _ _ w485 _ _ _ _ _]
      tunnel: w15 -> [_ _ _ _ w484 _ _ _ _ _]
      tunnel: w14 -> [_ _ _ _ w483 _ _ _ _ _]
      tunnel: w4 -> [_ _ _ _ _ _ _ _ _ _]
      tunnel: w13 -> [_ _ _ _ w482 _ _ _ _ _]
      tunnel: w12 -> [_ _ _ _ w481 _ _ _ _ _]
      tunnel: T2 {[], "Value"={"Q смещение"=0.0, "Q интервал"=0.0, "I смещение"=0.0, "I интервал"=0.0}, "Value"=[], "Value"=0} ("cluster") -> [_ _ _ w198 _ _ w895 _ _ _]
      event "Стоп": Value Change {
        n88 = event-data() -> ()  [unwired: 1 in, 1 out]
      }
      event "Интервалы и смещения.Q смещение", "Интервалы и смещения.Q интервал", "Интервалы и смещения.I смещение", "Интервалы и смещения.I интервал", "Точки карты (позиции)", "Соотношение точек с ПБ", "Все возможные точки карты", "Показать подписи точек на карте", "Смещение подписей.I", "Смещение подписей.Q", "Точки карты после разметки", "Количество каналов", "Цвет подписей точек": Value Change {
        w177 = u8 2 items=["По возрастанию", "По убыванию", "Пользовательское"] ("Соотношение точек с последовательностями битов")
        w163 = T3."Disabled and Grayed Out" ("Disabled")
        w164 = T3."Enabled" ("Disabled")
        n89 = event-data() -> ()  [unwired: 1 in, 1 out]
        n90 = Scale By Power Of 2(n="Количество каналов", x=ext 1.0) -> (x*2^n=→"Количество ПБ":ext)
        n91 = control-ref of="Перемешать соотношения"() -> (w166:refnum<vi>)
        n92 = Equal?(x="Соотношение точек с ПБ", y=w177) -> (x = y?=w165:bool)
        n93 = control-ref of="Точки карты (позиции)"() -> (w174:refnum<vi>)
        n94 = control-ref of="Размер карты (N*N)"() -> (w175:refnum<vi>)
        n95 = Select(t=w164, s=w165, f=T3."Disabled" ("Disabled")) -> (s? t:f=w171:T3)
        n96 = Select(t=w164, s=w165, f=w163) -> (s? t:f=w162:T3)
        n97 = Select(t=w163, s=w165, f=w164) -> (s? t:f=w173:T3)
        n98 = control-ref of="ПБ"() -> (w172:refnum<vi>)
        n99 = property class="Bool"(reference=w166, "DisabledEnum"=w162) -> ()  [unwired: 1 in, 2 out]
        n100 = property class="Slide (strict)"(reference=w175, "DisabledEnum"=w173) -> ()  [unwired: 1 in, 2 out]
        n101 = property class="Arr (strict)"(reference=w174, "DisabledEnum"=w173) -> ()  [unwired: 1 in, 2 out]
        n102 = property class="Ring (strict)"(reference=w172, "DisabledEnum"=w171) -> ()  [unwired: 1 in, 2 out]
      }
      event "Размер карты (N*N)": Value Change {
        n103 = event-data() -> ()  [unwired: 1 in, 1 out]
        n104 = control-ref of="Точки карты (позиции)"() -> (w179:refnum<vi>)
        n105 = feedback #1() -> (w178:i32)  [unwired: 1 in]
        n106 = feedback-in #1("Размер карты (N*N)") -> ()
        n107 = To Unsigned Long Integer(number="Размер карты (N*N)") -> (unsigned 32bit integer=w184:u32)
        n108 = property class="Arr (strict)"(reference=w179, "Number of Columns"=w184, "Number of Rows"=w184) -> ()  [unwired: 1 in, 2 out]
        n109 = property class="Arr (strict)"(reference=w179) -> ("Value"=w182:bool[][])  [unwired: 1 in, 2 out]
        n110 = Greater?(x="Размер карты (N*N)", y=w178) -> (0:w181:bool)
        n111 = case shown="False" w181 {
          tunnel: "Размер карты (N*N)" -> [w185 w190]
          tunnel: w182 -> [w187 w196]
          tunnel: [w186 w194] -> w183
          frame False {
            w188 = 0 ("index")
            n112 = Array Subset(array=w187, index (row)=w188, length (row)=w185, index (col)=w188, length (col)=w185) -> (w186:bool[][])
          }
          frame True {
            w197 = 0 ("index")
            n113 = Decrement(x=w190) -> (x-1=w191:i32)
            n114 = Array Subset(array=w196, index (row)=w197, length (row)=w191, index (col)=w197, length (col)=w191) -> (w195:bool[][])
            n115 = Initialize Array("Добавлять точки при\nувеличении размера карты", w190) -> (w193:bool[])
            n116 = Build Array (concatenate)(w195, w193) -> (w192:bool[][])
            n117 = Replace Array Subset(array=w192, new element=w193, index (col)=w191) -> (w194:bool[][])  [unwired: 1 in]
          }
        }
        n118 = property class="Arr (strict)"(reference=w179, "Value"=w183) -> ()  [unwired: 1 in, 2 out]
      }
      event "Загрузить карту из файла": Value Change {
        n119 = event-data() -> ()  [unwired: 1 in, 1 out]
        n120 = case shown="True" "Загрузить карту из файла" {
          tunnel: w198 -> [_ w225]
          frame False {
          }
          frame True {
            w201 = errorcluster {"status"=FALSE, "code"=0, "source"=""} ("error in (no error)")
            w205 = "[\\r\\n]*"
            n121 = call <vilib>:"Open_Create_Replace File.vi"("advisory dialog? (display:T)"=FALSE, "pattern"="*.xml", "prompt"="Выберите путь к XML файлу карты" ("Prompt"), "error in (no error)"=w201, "function (open:0)"=T4."open (read only)", "file path"="Путь для загрузки карты") -> ("error out"=w208:errorcluster, "file size (bytes)"=w209:i32, "refnum"=w210:refnum<file>)  [unwired: 2 in, 1 out]
            n122 = Concatenate Strings("</Version>", w205) -> (w214:string)
            n123 = Concatenate Strings(w205, "</LVData>" ("Substring")) -> (w215:string)
            n124 = Read from Binary File(8:w208, 10:w209, 11:w210) -> (0:w206:errorcluster, 2:w204:string, 3:w207:refnum<file>)  [unwired: 3 in, 1 out]
            n125 = control-ref of="Путь для загрузки карты"() -> (w232:refnum<vi>)
            n126 = Match Pattern(string=w204, regular expression=w214) -> (after substring=w216:string)  [unwired: 1 in, 3 out]
            n127 = Close File(refnum=w207, error in=w206) -> (path=w223:path, error out=w212:errorcluster)
            n128 = property class="Path"(reference=w232, "Value"=w223) -> ()  [unwired: 1 in, 2 out]
            n129 = Match Pattern(string=w216, regular expression=w215) -> (before substring=w213:string)  [unwired: 1 in, 3 out]
            n130 = case shown="No Error" w212 {
              selector: w212 -> [w247 w470]
              tunnel: w213 -> [w250 _]
              tunnel: string[] [] -> [w249 _]
              tunnel: [w248 string[] []] -> w211
              tunnel: w201 -> [w246 _]
              tunnel: [w245 w470] -> w200
              frame No Error {
                n131 = while {
                  shift-right: [w280] -> _
                  shift-left: w250 -> [w274]
                  shift-right: [w277] -> w248
                  shift-left: w249 -> [w278]
                  tunnel: w247 -> [w276]
                  tunnel: [w275] -> w245
                  tunnel: w246 -> [w251]
                  stop <- w279 stop-if-true
                  w252 = 1 ("offset (0)")
                  w253 = "<[A-Za-zАБВГДЕЖЗИЙКЛМНОПРСТУФХЦШЩЪЫЬЭЮЯабвгдежзийклмнопрстуфхцшщъыьэюя_:][A-Za-zАБВГДЕЖЗИЙКЛМНОПРСТУФХЦШЩЪЫЬЭЮЯабвгдежзийклмнопрстуфхцшщъыьэюя0-9\\.-_:·]*[\\t\\r\\n\\s]*>" ("Element")
                  w268 = 0 ("offset (0)")
                  n132 = Match Pattern(string=w274, regular expression=w253, offset (0)=w268) -> (before substring=w259:string, match substring=w260:string, after substring=w261:string, offset past match=w258:i32)
                  n133 = Match Pattern(string=w274, regular expression=w253, offset (0)=w268) -> (before substring=w263:string, match substring=w264:string, after substring=w265:string, offset past match=w262:i32)
                  n134 = String Subset(string=w260, offset (0)=w252) -> (substring=w257:string)  [unwired: 1 in]
                  n135 = String Subset(string=w264, offset (0)=w252) -> (substring=w255:string)  [unwired: 1 in]
                  n136 = Match Pattern(string=w257, regular expression="[\\t\\r\\n\\s]?>") -> (before substring=w267:string)  [unwired: 1 in, 3 out]
                  n137 = Match Pattern(string=w255, regular expression="[\\t\\r\\n\\s]?/>") -> (before substring=w266:string)  [unwired: 1 in, 3 out]
                  n138 = case shown="1, Default" w258 {
                    selector: w258 -> [_ w314]
                    tunnel: [w290 w316] -> w273
                    tunnel: w262 -> [w291 w315]
                    tunnel: w263 -> [w289 w310]
                    tunnel: w264 -> [w288 w309]
                    tunnel: w265 -> [w287 w308]
                    tunnel: w259 -> [_ w313]
                    tunnel: w260 -> [_ w312]
                    tunnel: w261 -> [_ w311]
                    tunnel: [w286 w307] -> w271
                    tunnel: [w285 w306] -> w270
                    tunnel: [w284 w305] -> w269
                    tunnel: w266 -> [w282 w304]
                    tunnel: w267 -> [_ w303]
                    tunnel: [w283 w302] -> w272
                    tunnel: [w281 w301] -> _
                    frame -1 {
                      n139 = case shown="1, Default" w291 {
                        selector: w291 -> [_ w296]
                        tunnel: [enum16{"Start Tag", "Empty Element", "Content"}."Content" enum16{"Start Tag", "Empty Element", "Content"}."Empty Element"] -> w290
                        tunnel: w289 -> [_ w300]
                        tunnel: w288 -> [_ w299]
                        tunnel: w287 -> [_ w298]
                        tunnel: [w294 w300] -> w286
                        tunnel: [w294 w299] -> w285
                        tunnel: [w294 w298] -> w284
                        tunnel: [w294 w297] -> w283
                        tunnel: w282 -> [_ w297]
                        tunnel: [-1 ("offset past match") w296] -> w281
                        frame -1 {
                          w294 = ""
                        }
                        frame 1, Default {
                        }
                      }
                    }
                    frame 1, Default {
                      n140 = case shown="1, Default" w315 {
                        selector: w315 -> [_ w336]
                        tunnel: [enum16{"Start Tag", "Empty Element", "Content"}."Start Tag" w339] -> w316
                        tunnel: w314 -> [w318 w337]
                        tunnel: w313 -> [w322 w335]
                        tunnel: w312 -> [w321 w334]
                        tunnel: w311 -> [w320 w333]
                        tunnel: w310 -> [_ w332]
                        tunnel: w309 -> [_ w331]
                        tunnel: w308 -> [_ w330]
                        tunnel: [w322 w329] -> w307
                        tunnel: [w321 w328] -> w306
                        tunnel: [w320 w327] -> w305
                        tunnel: w304 -> [_ w326]
                        tunnel: w303 -> [w319 w324]
                        tunnel: [w319 w325] -> w302
                        tunnel: [w318 w323] -> w301
                        frame -1 {
                        }
                        frame 1, Default {
                          n141 = Greater?(x=w337, y=w336) -> (0:w338:bool)
                          n142 = case shown="True" w338 {
                            tunnel: [enum16{"Start Tag", "Empty Element", "Content"}."Start Tag" enum16{"Start Tag", "Empty Element", "Content"}."Empty Element"] -> w339
                            tunnel: w337 -> [w341 _]
                            tunnel: w336 -> [_ w347]
                            tunnel: w335 -> [w345 _]
                            tunnel: w334 -> [w344 _]
                            tunnel: w333 -> [w343 _]
                            tunnel: w332 -> [_ w351]
                            tunnel: w331 -> [_ w350]
                            tunnel: w330 -> [_ w349]
                            tunnel: [w345 w351] -> w329
                            tunnel: [w344 w350] -> w328
                            tunnel: [w343 w349] -> w327
                            tunnel: w326 -> [_ w348]
                            tunnel: [w342 w348] -> w325
                            tunnel: w324 -> [w342 _]
                            tunnel: [w341 w347] -> w323
                            frame False {
                            }
                            frame True {
                            }
                          }
                        }
                      }
                    }
                  }
                  n143 = case shown="\"Start Tag\"" w273 {
                    tunnel: [w365 w461 ""] -> w280
                    tunnel: [w359 FALSE TRUE] -> w279
                    tunnel: w278 -> [w367 w465 w466]
                    tunnel: [w363 w463 w466] -> w277
                    tunnel: w276 -> [w369 w462 w469]
                    tunnel: [w364 w462 w469] -> w275
                    tunnel: w272 -> [w370 _ _]
                    tunnel: w271 -> [_ _ _]
                    tunnel: w270 -> [w366 w464 _]
                    tunnel: w269 -> [w371 w461 _]
                    tunnel: w251 -> [w352 _ _]
                    frame "Start Tag" {
                      n144 = while {
                        tunnel: w371 -> [w379]
                        tunnel: w370 -> [w377]
                        shift-right: [w375] -> w368
                        shift-left: w369 -> [w387]
                        shift-right: [w382] -> w358
                        shift-left: 0 ("offset past match") -> [w384]
                        shift-right: [w380] -> _
                        shift-left: 1 ("offset past match") -> [w386]
                        tunnel: [w378] -> w361
                        tunnel: [w379] -> w356
                        tunnel: w352 -> [w372]
                        stop <- w376 stop-if-true
                        w373 = "[\\t\\r\\n\\s]*>" ("regular expression")
                        n145 = case shown="1, Default" w384 {
                          selector: w384 -> [w401 w404]
                          tunnel: [w400 w408] -> _
                          tunnel: [w400 w407] -> _
                          tunnel: [w401 w406] -> w383
                          tunnel: [w400 w405] -> _
                          tunnel: w377 -> [_ w403]
                          tunnel: w379 -> [_ w410]
                          tunnel: w373 -> [_ w402]
                          frame -1 {
                            w400 = ""
                          }
                          frame 1, Default {
                            n146 = Concatenate Strings("<" ("left angle"), w403, w402) -> (w409:string)
                            n147 = Match Pattern(string=w410, regular expression=w409, offset (0)=w404) -> (before substring=w408:string, match substring=w405:string, after substring=w407:string, offset past match=w406:i32)
                          }
                        }
                        n148 = case shown="1, Default" w384 {
                          selector: w384 -> [w389 w394]
                          tunnel: w379 -> [_ w399]
                          tunnel: w377 -> [_ w392]
                          tunnel: [w388 w398] -> _
                          tunnel: [w388 w397] -> w378
                          tunnel: [w388 w396] -> _
                          tunnel: [w389 w395] -> w385
                          tunnel: w373 -> [_ w390]
                          frame -1 {
                            w388 = ""
                          }
                          frame 1, Default {
                            n149 = Concatenate Strings("</" ("string"), w392, w390) -> (w391:string)
                            n150 = Match Pattern(string=w399, regular expression=w391, offset (0)=w394) -> (before substring=w398:string, match substring=w397:string, after substring=w396:string, offset past match=w395:i32)
                          }
                        }
                        n151 = case shown="-1" w385 {
                          selector: w385 -> [_ w429]
                          tunnel: w383 -> [_ w426]
                          tunnel: [0 ("offset past match") w430] -> w382
                          tunnel: w386 -> [w424 w428]
                          tunnel: [w423 w427] -> w380
                          tunnel: w387 -> [_ w425]
                          tunnel: [w421 w425] -> w375
                          tunnel: w377 -> [w415 _]
                          tunnel: w372 -> [w412 _]
                          frame -1 {
                            n152 = Decrement(x=w424) -> (x-1=w423:i32)
                            n153 = Current VI's Path() -> (path=w413:path)
                            n154 = Strip Path(path=w413) -> (name=w419:string)  [unwired: 1 out]
                            n155 = Concatenate Strings(w419, "<append>----\n" ("string"), "End tag not found\nfor <" ("error message"), w415, ">" ("string")) -> (w417:string)
                            n156 = Bundle By Name(cluster=w412, "source"=w417, "status"=TRUE) -> (w421:errorcluster)
                          }
                          frame 1, Default {
                            n157 = case shown="1, Default" w426 {
                              selector: w426 -> [_ w434]
                              tunnel: [w431 w438] -> w430
                              tunnel: w429 -> [w431 w437]
                              tunnel: w428 -> [w433 w436]
                              tunnel: [w432 w435] -> w427
                              frame -1 {
                                n158 = Decrement(x=w433) -> (x-1=w432:i32)
                              }
                              frame 1, Default {
                                n159 = Greater?(x=w434, y=w437) -> (0:w439:bool)
                                n160 = case shown="False" w439 {
                                tunnel: w437 -> [_ w443]
                                tunnel: w434 -> [w440 _]
                                tunnel: [w440 w443] -> w438
                                tunnel: w436 -> [w442 w445]
                                tunnel: [w441 w444] -> w435
                                frame False {
                                n161 = Increment(x=w442) -> (x+1=w441:i32)
                                }
                                frame True {
                                n162 = Decrement(x=w445) -> (x-1=w444:i32)
                                }
                                }
                              }
                            }
                          }
                        }
                        n163 = Unbundle By Name(w375) -> ("status"=w374:bool)
                        n164 = Equal To 0?(x=w380) -> (x = 0?=w381:bool)
                        n165 = Or(x=w374, y=w381) -> (x .or. y?=w376:bool)
                      }
                      n166 = String Length(string=w361) -> (length=w357:i32)
                      n167 = String Subset(string=w356, offset (0)=w358) -> (substring=w360:string)  [unwired: 1 in]
                      n168 = Subtract(x=w358, y=w357) -> (x-y=w355:i32)
                      n169 = String Subset(string=w356, length (rest)=w355) -> (substring=w362:string)  [unwired: 1 in]
                      n170 = case shown="No Error" w368 {
                        selector: w368 -> [w453 w459]
                        tunnel: w362 -> [w454 _]
                        tunnel: w367 -> [w451 _]
                        tunnel: w366 -> [w455 _]
                        tunnel: [w448 ""] -> w365
                        tunnel: [w453 w459] -> w364
                        tunnel: [w450 string[] []] -> w363
                        tunnel: w361 -> [w449 _]
                        tunnel: w360 -> [w448 _]
                        tunnel: [FALSE TRUE] -> w359
                        frame No Error {
                          n171 = Concatenate Strings(w455, w454, w449, "\r\n") -> (w452:string)
                          n172 = Build Array (concatenate)(w451, w452) -> (w450:string[])
                        }
                        frame Error {
                          # "no matching close tag found"
                        }
                      }
                    }
                    frame "Empty Element" {
                      n173 = Build Array (concatenate)(w465, w464) -> (w463:string[])
                    }
                    frame "Content" {
                    }
                  }
                }
              }
              frame Error {
              }
            }
            n174 = case shown="No Error" w200 {
              frame No Error {
                n175 = One Button Dialog(message="Карта успешно загружена.") -> ()  [unwired: 1 in, 1 out]
              }
              frame Error {
                n176 = call <vilib>:"General Error Handler.vi"() -> ("error?"=w244:bool)  [unwired: 11 in, 4 out]
                n177 = Stop(stop? (T)=w244) -> ()
              }
            }
            n178 = Concatenate Strings(w211) -> (w222:string)
            n179 = control-ref of="Все возможные точки карты"() -> (w234:refnum<vi>)
            n180 = control-ref of="Соотношение точек с ПБ"() -> (w227:refnum<vi>)
            n181 = control-ref of="Интервалы и смещения"() -> (w235:refnum<vi>)
            n182 = Unflatten From XML(xml string=w222, type=w225) -> (value=w231:T2)  [unwired: 1 in, 1 out]
            n183 = Unbundle(w231) -> (w230:i16[][], "Value"=w229:T1, "Value"=w228:cluster{"I":dbl, "Q":dbl, "Биты":u32}[], "Value"=w226:u8)
            n184 = control-ref of="Размер карты (N*N)"() -> (w237:refnum<vi>)
            n185 = Array Size(array=w230) -> (size(s)=w242:i32[])
            n186 = property class="Clust (strict)"(reference=w235, "Value"=w229) -> ()  [unwired: 1 in, 2 out]
            n187 = property class="Arr (strict)"(reference=w234, "Value"=w228) -> ()  [unwired: 1 in, 2 out]
            n188 = property class="Ring (strict)"(reference=w227, "Value"=w226) -> ()  [unwired: 1 in, 2 out]
            n189 = Index Array(array=w242) -> (element=w239:i32)  [unwired: 1 in]
            n190 = property class="Slide (strict)"(reference=w237, "Value"=w239) -> ("Value"=w233:i32)  [unwired: 1 in, 2 out]
            n191 = for {
              N: w239 -> [w474]
              tunnel: w230 -> [w473] mode=indexing
              tunnel: [w472] -> w241 mode=indexing
              n192 = for {
                N: w474 -> [_]
                tunnel: w473 -> [w476] mode=indexing
                tunnel: [w477] -> w472 mode=indexing
                n193 = Greater Than 0?(x=w476) -> (x > 0?=w475:bool)
                n194 = Select(t=TRUE, s=w475, f=FALSE) -> (s? t:f=w477:bool)
              }
            }
            n195 = control-ref of="Точки карты (позиции)"() -> (w236:refnum<vi>)
            n196 = To Unsigned Long Integer(number=w233) -> (unsigned 32bit integer=w238:u32)
            n197 = To Unsigned Long Integer(number=w239) -> (unsigned 32bit integer=w240:u32)
            n198 = property class="Arr (strict)"(reference=w236, "Number of Columns"=w238, "Number of Rows"=w238) -> ()  [unwired: 1 in, 2 out]
            n199 = property class="Arr (strict)"(reference=w236, "Number of Columns"=w240, "Number of Rows"=w240, "Value"=w241) -> ()  [unwired: 1 in, 2 out]
          }
        }
      }
      event "Построить карту с помощью разметки": Value Change {
        n200 = event-data() -> ()  [unwired: 1 in, 1 out]
        n201 = case shown="True" "Построить карту с помощью разметки" {
          tunnel: w486 -> [_ w516]
          tunnel: w485 -> [_ w515]
          tunnel: w484 -> [_ w514]
          tunnel: w483 -> [_ w513]
          tunnel: w482 -> [_ w512]
          tunnel: w481 -> [_ w511]
          frame False {
          }
          frame True {
            w487 = u16 1 items=["unsigned binary", "offset binary", "2's complement"] ("data format (offset binary)")
            w488 = 2.0 ("full-scale range (pk-pk)")
            w489 = errorcluster {"status"=FALSE, "code"=0, "source"=""} ("error in (no error)")
            n202 = case shown="1" "Источник БП" {
              tunnel: [w629 w649] -> w497
              tunnel: w489 -> [_ w647]
              tunnel: w488 -> [_ w646]
              tunnel: w487 -> [_ w645]
              frame 0, Default {
                n203 = control-ref of="Количество каналов"() -> (w632:refnum<vi>)
                n204 = property class="DigNum (strict)"(reference=w632) -> ("Value"=w631:i32)  [unwired: 1 in, 2 out]
                n205 = To Long Integer(number="Частота дискретизации случайной последовательности") -> (32bit integer=w634:i32)
                n206 = Reciprocal(x="Частота дискретизации случайной последовательности") -> (1/x=w635:dbl)
                n207 = for {
                  N: w634 -> [_]
                  tunnel: [w638] -> w633 mode=indexing
                  tunnel: w631 -> [w637]
                  n208 = for {
                    N: w637 -> [_]
                    tunnel: [w642] -> w638 mode=indexing
                    n209 = Random Number (0-1)() -> (number: 0 to 1=w639:dbl)
                    n210 = Round To Nearest(number=w639) -> (nearest integer value=w640:dbl)
                    n211 = Greater Than 0?(x=w640) -> (x > 0?=w641:bool)
                    n212 = Select(t=u8 1, s=w641, f=u8 0) -> (s? t:f=w642:u8)
                  }
                }
                n213 = Bundle By Name("data"=w633) -> (w630:digitaldata)  [unwired: 1 in]
                n214 = Bundle By Name("dt"=w635, "Y"=w630) -> (w629:digitalwaveform)  [unwired: 1 in]
              }
              frame 1 {
                n215 = control-ref of="Путь к wav файлу"() -> (w656:refnum<vi>)
                n216 = call <vilib>:"Sound File Read Simple.vi"("path"="Путь к wav файлу") -> ("data"=w654:waveform(dbl)[], "path out"=w655:path)  [unwired: 7 in, 2 out]
                n217 = property class="Path"(reference=w656, "Value"=w655) -> ()  [unwired: 1 in, 2 out]
                n218 = call "Convert to Dynamic Data2"("Array of Waveforms"=w654) -> ("Dynamic Data Type"=w651:dynamicdata)  [unwired: 3 in]
                n219 = call "Convert from Dynamic Data"("Dynamic Data Type"=w651, "Channel"=0) -> ("Waveform"=w653:waveform(dbl))  [unwired: 2 in]
                n220 = case shown="No Error" w647 {
                  selector: w647 -> [w672 w861]
                  tunnel: w653 -> [w673 _]
                  tunnel: [w677 _] -> w649
                  tunnel: [w666 w861] -> _
                  tunnel: "глубина кодирования (бит)" -> [w671 w860]
                  tunnel: FALSE ("compress digital (T)") -> [w670 _]
                  tunnel: w645 -> [w669 _]
                  tunnel: [w667 w860] -> _
                  tunnel: w646 -> [w665 w859]
                  tunnel: [w665 w859] -> _
                  frame No Error {
                    w664 = u16 2 items=["Unsigned Binary", "Offset Binary", "2's Compliment"] ("data format (offset binary)")
                    n221 = Equal?(x=w669, y=w664) -> (x = y?=w663:bool)
                    n222 = Select(t=2 ("lower limit"), s=w663, f=1 ("lower limit")) -> (s? t:f=w662:i32)
                    n223 = In Range and Coerce(upper limit=54, x=w671, lower limit=w662) -> (coerced(x)=w667:i32, In Range?=w659:bool)
                    n224 = case shown="No Error" w672 {
                      selector: w672 -> [_ w858]
                      tunnel: w673 -> [w690 _]
                      tunnel: [w685 _] -> w668
                      tunnel: w667 -> [w688 _]
                      tunnel: [w681 w858] -> w666
                      tunnel: w659 -> [w689 _]
                      tunnel: w665 -> [w679 _]
                      tunnel: w670 -> [w684 _]
                      tunnel: w669 -> [w683 _]
                      frame No Error {
                        n225 = Greater Than 0?(x=w679) -> (x > 0?=w678:bool)
                        n226 = case shown="True" w678 {
                          tunnel: w690 -> [_ w705]
                          tunnel: w689 -> [_ w702]
                          tunnel: w688 -> [_ w698]
                          tunnel: [_ w695] -> w687
                          tunnel: w683 -> [_ w694]
                          tunnel: [-1816 ("f") w693] -> w682
                          tunnel: w679 -> [_ w692]
                          frame False {
                          }
                          frame True {
                            n227 = Unbundle By Name(w705) -> ("Y"=w697:dbl[])
                            n228 = Select(t=0, s=w702, f=1809) -> (s? t:f=w696:i32)
                            n229 = Array Size(array=w697) -> (size(s)=w701:i32)
                            n230 = Initialize Array(u8 0, w701, w698) -> (w699:u8[][])
                            n231 = case shown="2" w694 {
                              tunnel: w692 -> [w706 w754 w803]
                              tunnel: w699 -> [w718 w765 w814]
                              tunnel: w697 -> [w717 w764 w813]
                              tunnel: w698 -> [w708 w751 w800]
                              tunnel: w696 -> [w712 w760 w809]
                              tunnel: [w711 w759 w808] -> w695
                              tunnel: [w710 w758 w807] -> w693
                              frame 0, Default {
                                n232 = Scale By Power Of 2(n=w708, x=1.0) -> (x*2^n=w707:dbl)
                                n233 = Divide(x=w706, y=w707) -> (x/y=w716:dbl)
                                n234 = for {
                                shift-right: [w727] -> w711
                                shift-left: w718 -> [w728]
                                tunnel: w717 -> [w719] mode=indexing
                                tunnel: w716 -> [w724]
                                shift-right: [w725] -> w714
                                shift-left: FALSE ("f") -> [w721]
                                tunnel: w708 -> [w723]
                                i -> [w726]
                                n235 = Divide(x=w719, y=w724) -> (x/y=w729:dbl)
                                n236 = Decrement(x=w723) -> (x-1=w722:i32)
                                n237 = Not A Number/Path/Refnum?(number/path/refnum=w719) -> (NaN/Path/Refnum?=w720:bool)
                                n238 = Or(x=w721, y=w720) -> (x .or. y?=w725:bool)
                                n239 = for {
                                N: w723 -> [_]
                                shift-right: [w734] -> _
                                shift-left: w729 -> [w735]
                                tunnel: w722 -> [w740]
                                shift-right: [w737] -> w727
                                shift-left: w728 -> [w738]
                                tunnel: w726 -> [w736]
                                i -> [w730]
                                n240 = Subtract(x=w740, y=w730) -> (x-y=w731:i32)
                                n241 = Scale By Power Of 2(n=w731, x=1.0) -> (x*2^n=w732:dbl)
                                n242 = Greater Or Equal?(x=w735, y=w732) -> (x >= y?=w739:bool)
                                n243 = case shown="True" w739 {
                                tunnel: w738 -> [w741 w750]
                                tunnel: [w741 w749] -> w737
                                tunnel: w730 -> [_ w748]
                                tunnel: w736 -> [_ w747]
                                tunnel: w735 -> [w742 w745]
                                tunnel: w732 -> [_ w744]
                                tunnel: [w742 w743] -> w734
                                frame False {
                                }
                                frame True {
                                n244 = Subtract(x=w745, y=w744) -> (x-y=w743:dbl)
                                n245 = Replace Array Subset(array=w750, new element=u8 1 ("New Element/Subarray"), index (row)=w747, index (col)=w748) -> (w749:u8[][])
                                }
                                }
                                }
                                }
                                n246 = Select(t=-1804, s=w714, f=w712) -> (s? t:f=w710:i32)
                              }
                              frame 1 {
                                # "FS/2"
                                # "LSB"
                                n247 = Scale By Power Of 2(n=w751, x=1.0) -> (x*2^n=w756:dbl)
                                n248 = Divide(x=w754, y=2.0) -> (x/y=w752:dbl)
                                n249 = Divide(x=w754, y=w756) -> (x/y=w755:dbl)
                                n250 = for {
                                shift-right: [w766] -> w759
                                shift-left: w765 -> [w778]
                                tunnel: w764 -> [w770] mode=indexing
                                tunnel: w755 -> [w769]
                                shift-right: [w777] -> w762
                                shift-left: FALSE ("f") -> [w775]
                                tunnel: w751 -> [w772]
                                tunnel: w752 -> [w771]
                                i -> [w773]
                                n251 = Add(x=w770, y=w771) -> (x+y=w768:dbl)
                                n252 = Not A Number/Path/Refnum?(number/path/refnum=w770) -> (NaN/Path/Refnum?=w774:bool)
                                n253 = Divide(x=w768, y=w769) -> (x/y=w767:dbl)
                                n254 = Or(x=w775, y=w774) -> (x .or. y?=w777:bool)
                                n255 = Decrement(x=w772) -> (x-1=w776:i32)
                                n256 = for {
                                N: w772 -> [_]
                                shift-right: [w783] -> _
                                shift-left: w767 -> [w784]
                                tunnel: w776 -> [w789]
                                shift-right: [w786] -> w766
                                shift-left: w778 -> [w787]
                                tunnel: w773 -> [w785]
                                i -> [w779]
                                n257 = Subtract(x=w789, y=w779) -> (x-y=w780:i32)
                                n258 = Scale By Power Of 2(n=w780, x=1.0) -> (x*2^n=w781:dbl)
                                n259 = Greater Or Equal?(x=w784, y=w781) -> (x >= y?=w788:bool)
                                n260 = case shown="True" w788 {
                                tunnel: w787 -> [w790 w799]
                                tunnel: [w790 w798] -> w786
                                tunnel: w779 -> [_ w797]
                                tunnel: w785 -> [_ w796]
                                tunnel: w784 -> [w791 w794]
                                tunnel: w781 -> [_ w793]
                                tunnel: [w791 w792] -> w783
                                frame False {
                                }
                                frame True {
                                n261 = Subtract(x=w794, y=w793) -> (x-y=w792:dbl)
                                n262 = Replace Array Subset(array=w799, new element=u8 1 ("New Element/Subarray"), index (row)=w796, index (col)=w797) -> (w798:u8[][])
                                }
                                }
                                }
                                }
                                n263 = Select(t=-1804, s=w762, f=w760) -> (s? t:f=w758:i32)
                              }
                              frame 2 {
                                n264 = Scale By Power Of 2(n=w800, x=1.0) -> (x*2^n=w805:dbl)
                                n265 = Divide(x=w803, y=w805) -> (x/y=w804:dbl)
                                n266 = Divide(x=w803, y=2.0) -> (x/y=w801:dbl)
                                n267 = for {
                                shift-right: [w815] -> w808
                                shift-left: w814 -> [w827]
                                tunnel: w813 -> [w819] mode=indexing
                                tunnel: w804 -> [w818]
                                shift-right: [w826] -> w811
                                shift-left: FALSE ("f") -> [w824]
                                tunnel: w800 -> [w821]
                                tunnel: w801 -> [w820]
                                i -> [w822]
                                n268 = Add(x=w819, y=w820) -> (x+y=w817:dbl)
                                n269 = Not A Number/Path/Refnum?(number/path/refnum=w819) -> (NaN/Path/Refnum?=w823:bool)
                                n270 = Divide(x=w817, y=w818) -> (x/y=w816:dbl)
                                n271 = Or(x=w824, y=w823) -> (x .or. y?=w826:bool)
                                n272 = Decrement(x=w821) -> (x-1=w825:i32)
                                n273 = for {
                                N: w821 -> [_]
                                shift-right: [w835] -> _
                                shift-left: w816 -> [w836]
                                tunnel: w825 -> [w840]
                                shift-right: [w838] -> w815
                                shift-left: w827 -> [w839]
                                tunnel: w822 -> [w837]
                                i -> [w830]
                                n274 = Subtract(x=w840, y=w830) -> (x-y=w831:i32)
                                n275 = Scale By Power Of 2(n=w831, x=1.0) -> (x*2^n=w833:dbl)
                                n276 = Equal To 0?(x=w830) -> (x = 0?=w832:bool)
                                n277 = Greater Or Equal?(x=w836, y=w833) -> (x >= y?=w829:bool)
                                n278 = case shown="True" w829 {
                                tunnel: w836 -> [w847 w850]
                                tunnel: [w847 w849] -> w835
                                tunnel: w833 -> [_ w848]
                                frame False {
                                }
                                frame True {
                                n279 = Subtract(x=w850, y=w848) -> (x-y=w849:dbl)
                                }
                                }
                                n280 = Exclusive Or(1:w832, 2:w829) -> (0:w828:bool)
                                n281 = case shown="True" w828 {
                                tunnel: w839 -> [w841 w846]
                                tunnel: [w841 w845] -> w838
                                tunnel: w837 -> [_ w844]
                                tunnel: w830 -> [_ w843]
                                frame False {
                                }
                                frame True {
                                n282 = Replace Array Subset(array=w846, new element=u8 1 ("New Element/Subarray"), index (row)=w844, index (col)=w843) -> (w845:u8[][])
                                }
                                }
                                }
                                }
                                n283 = Select(t=-1804, s=w811, f=w809) -> (s? t:f=w807:i32)
                              }
                            }
                          }
                        }
                        n284 = Greater Or Equal To 0?(x=w682) -> (x >= 0?=w686:bool)
                        n285 = case shown="True" w686 {
                          tunnel: [_ w854] -> w685
                          tunnel: w687 -> [_ w852]
                          tunnel: w684 -> [_ w851]
                          frame False {
                          }
                          frame True {
                            n286 = Bundle By Name("data"=w852) -> (w853:digitaldata)  [unwired: 1 in]
                            n287 = case shown="True" w851 {
                              tunnel: [w855 w857] -> w854
                              tunnel: w853 -> [w855 w856]
                              frame False {
                              }
                              frame True {
                                n288 = call <vilib>:"DTbl Compress Digital.vi"("uncompressed digital data"=w856) -> ("compressed digital data"=w857:digitaldata)  [unwired: 9 in, 1 out]
                              }
                            }
                          }
                        }
                        n289 = call <vilib>:"Error Cluster From Error Code.vi"("show call chain? (False)"=TRUE, "error code (0)"=w682) -> ("error out"=w681:errorcluster)  [unwired: 7 in]
                      }
                      frame Error {
                      }
                    }
                    n290 = Unbundle By Name(w673) -> ("attributes"=w675:variant, "t0"=w674:timestamp, "dt"=w676:dbl)
                    n291 = Bundle By Name("attributes"=w675, "t0"=w674, "dt"=w676, "Y"=w668) -> (w677:digitalwaveform)  [unwired: 1 in]
                  }
                  frame Error {
                    # "Return empty array\non input error."
                  }
                }
              }
            }
            "Временная диаграмма каналов" <- w497
            "digital waveform" <- w497
            n292 = control-ref of="Все возможные точки карты"() -> (w508:refnum<vi>)
            n293 = property class="Arr (strict)"(reference=w508) -> ("Value"=w499:cluster{"I":dbl, "Q":dbl, "ПБ":u32}[])  [unwired: 1 in, 2 out]
            n294 = control-ref of="Цвет подписей точек"() -> (w496:refnum<vi>)
            n295 = for {
              tunnel: w499 -> [w628] mode=indexing
              tunnel: [w627] -> w503 mode=indexing
              n296 = Unbundle By Name(w628) -> ("ПБ"=w627:u32)
            }
            n297 = case shown="True" "Воспроизвести" {
              tunnel: w497 -> [_ w529]
              tunnel: w489 -> [_ w527]
              tunnel: w488 -> [_ w526]
              tunnel: w487 -> [_ w525]
              frame False {
              }
              frame True {
                n298 = case shown="No Error" w527 {
                  selector: w527 -> [w536 w608]
                  tunnel: [w535 w608] -> _
                  tunnel: [w542 w607] -> w528
                  tunnel: w529 -> [w541 _]
                  tunnel: [w534 _] -> _
                  tunnel: w526 -> [w532 w603]
                  tunnel: [w532 w603] -> _
                  tunnel: w525 -> [w531 _]
                  frame No Error {
                    n299 = Unbundle By Name(w541) -> ("attributes"=w538:variant, "t0"=w539:timestamp, "dt"=w540:dbl, "Y"=w537:digitaldata)
                    n300 = case shown="No Error" w536 {
                      selector: w536 -> [w548 w602]
                      tunnel: [w547 w602] -> w535
                      tunnel: [w550 w601] -> w533
                      tunnel: w537 -> [w549 _]
                      tunnel: w532 -> [w544 _]
                      tunnel: w531 -> [w546 _]
                      tunnel: [w545 _] -> w534
                      frame No Error {
                        n301 = Greater Than 0?(x=w544) -> (x > 0?=w543:bool)
                        n302 = case shown="True" w543 {
                          tunnel: [_ w564] -> w550
                          tunnel: w549 -> [_ w563]
                          tunnel: w548 -> [w553 w562]
                          tunnel: [w551 w555] -> w547
                          tunnel: w546 -> [_ w561]
                          tunnel: w544 -> [_ w560]
                          tunnel: [_ w557] -> w545
                          frame False {
                            n303 = call <vilib>:"Error Cluster From Error Code.vi"("show call chain? (False)"=TRUE, "error in (no error)"=w553, "error code (0)"=-1816) -> ("error out"=w551:errorcluster)  [unwired: 6 out]
                          }
                          frame True {
                            n304 = call-poly <vilib>:"Digital Size.vi"("error in (no error)"=w562, "digital data in"=w563) -> ("error out"=w555:errorcluster, "number of signals"=w557:i32, "number of samples"=w559:i32, "digital data out"=w556:digitaldata)  [unwired: 6 out]
                            n305 = case shown="2" w561 {
                              tunnel: w560 -> [w570 w581 w593]
                              tunnel: w559 -> [_ _ _]
                              tunnel: w556 -> [w568 w577 w589]
                              tunnel: w557 -> [w567 w576 w585]
                              tunnel: [w566 w578 w590] -> w558
                              frame 0, Default {
                                n306 = Scale By Power Of 2(n=w567, x=1.0) -> (x*2^n=w571:dbl)
                                n307 = Divide(x=w570, y=w571) -> (x/y=w569:dbl)
                                n308 = call <vilib>:"Generate Value.vi"("Digital data in"=w568) -> ("Analog Data"=w565:dbl[])  [unwired: 2 in, 8 out]
                                n309 = Multiply(x=w565, y=w569) -> (x*y=w566:dbl[])
                              }
                              frame 1 {
                                # "LSB"
                                n310 = Scale By Power Of 2(n=w576, x=1.0) -> (x*2^n=w582:dbl)
                                n311 = Divide(x=w581, y=w582) -> (x/y=w575:dbl)
                                n312 = Divide(x=w581, y=2.0) -> (x/y=w579:dbl)
                                n313 = call <vilib>:"Generate Value.vi"("Digital data in"=w577) -> ("Analog Data"=w573:dbl[])  [unwired: 2 in, 8 out]
                                n314 = Multiply(x=w573, y=w575) -> (x*y=w574:dbl[])
                                n315 = Subtract(x=w574, y=w579) -> (x-y=w578:dbl[])
                              }
                              frame 2 {
                                n316 = Decrement(x=w585) -> (x-1=w587:i32)
                                n317 = Scale By Power Of 2(n=w585, x=1.0) -> (x*2^n=w595:dbl)
                                n318 = Divide(x=w593, y=w595) -> (x/y=w596:dbl)
                                n319 = call-poly <vilib>:"Invert Digital.vi"("number of signals (-1:all)"=1, "signal index (0)"=w587, "digital data"=w589) -> ("inverted digital data"=w588:digitaldata)  [unwired: 2 in, 6 out]
                                n320 = call <vilib>:"Generate Value.vi"("Digital data in"=w588) -> ("Analog Data"=w584:dbl[])  [unwired: 2 in, 8 out]
                                n321 = Multiply(x=w584, y=w596) -> (x*y=w594:dbl[])
                                n322 = Divide(x=w593, y=2.0) -> (x/y=w591:dbl)
                                n323 = Subtract(x=w594, y=w591) -> (x-y=w590:dbl[])
                              }
                            }
                            n324 = Bundle By Name("Y"=w558) -> (w564:waveform(dbl))  [unwired: 1 out]
                          }
                        }
                      }
                      frame Error {
                        w600 = 0.0 ("t0")
                        n325 = To Time Stamp(1:w600) -> (0:w598:timestamp)
                        n326 = Bundle By Name("t0"=w598, "dt"=w600, "Y"=dbl[] []) -> (w601:waveform(dbl))  [unwired: 1 out]
                      }
                    }
                    n327 = Bundle By Name(cluster=w533, "attributes"=w538, "t0"=w539, "dt"=w540) -> (w542:waveform(dbl))
                  }
                  frame Error {
                    w606 = 0.0 ("t0")
                    n328 = To Time Stamp(1:w606) -> (0:w604:timestamp)
                    n329 = Bundle By Name("t0"=w604, "dt"=w606, "Y"=dbl[] []) -> (w607:waveform(dbl))  [unwired: 1 in]
                  }
                }
                n330 = call "Convert to Dynamic Data"("Waveform"=w528) -> ("Dynamic Data Type"=w530:dynamicdata)  [unwired: 3 in]
                n331 = call "Play Waveform"("Data"=w530) -> ()  [unwired: 18 in, 1 out]
              }
            }
            n332 = Unbundle By Name(w497) -> ("Y"=w509:digitaldata)
            n333 = property class="ColBox"(reference=w496) -> ("Value"=w495:u32)  [unwired: 1 in, 2 out]
            n334 = call-poly <vilib>:"Digital to Binary.vi"("digital data"=w509) -> ("binary array"=w502:u32[])  [unwired: 9 in, 1 out]
            n335 = for {
              tunnel: [w626] -> w491 mode=indexing
              tunnel: w512 -> [w625]
              tunnel: w511 -> [w624]
              tunnel: w495 -> [w623]
              tunnel: w514 -> [w622]
              tunnel: w513 -> [w621]
              tunnel: "%b" ("format string") -> [w620]
              tunnel: w503 -> [w611]
              tunnel: w502 -> [w610] mode=indexing
              tunnel: w499 -> [w618]
              tunnel: w516 -> [w617]
              tunnel: [w616] -> w501 mode=indexing
              tunnel: [w612] -> w500 mode=indexing
              n336 = Search 1D Array(1D array=w611, element=w610) -> (index of element=w609:i32)  [unwired: 1 in]
              n337 = Index Array(array=w618, index=w609) -> (element=w612:cluster{"I":dbl, "Q":dbl, "ПБ":u32})
              n338 = Unbundle By Name(w612) -> ("I"=w614:dbl, "Q"=w613:dbl, "ПБ"=w615:u32)
              n339 = Bundle By Name(cluster=w617, "I"=w614, "Q"=w613) -> (w616:cluster{"I":dbl, "Q":dbl})
              n340 = Format Into String(format string=w620, w615) -> (resulting string=w619:string)  [unwired: 2 in, 1 out]
              n341 = Bundle By Name(cluster=w622, "Position.X"=w614, "Position.Y"=w613, "Name"=w619, "Lock Name"=w621, "Name Visible"=w624, "Label Offset"=w625, "Color"=w623) -> (w626:T5)
            }
            n342 = control-ref of="Точки карты после разметки"() -> (w507:refnum<vi>)
            n343 = Build Cluster Array(w501, w515) -> (→"Карта 2":cluster{cluster{"I":dbl, "Q":dbl}[]}[])
            n344 = property class="Arr (strict)"(reference=w507, "Value"=w500) -> ()  [unwired: 1 in, 2 out]
            n345 = Index Array(array=w491) -> (element=w492:T5)  [unwired: 1 in]
            n346 = Initialize Array(w492, 0 ("Dimension Size")) -> (w493:T6)
            n347 = for {
              tunnel: w491 -> [w519] mode=indexing
              shift-right: [w518] -> w490
              shift-left: w493 -> [w517]
              n348 = Search 1D Array(1D array=w517, element=w519) -> (index of element=w520:i32)  [unwired: 1 in]
              n349 = case shown="-1" w520 {
                tunnel: w519 -> [_ w524]
                tunnel: [w521 w522] -> w518
                tunnel: w517 -> [w521 w523]
                frame Default {
                }
                frame -1 {
                  n350 = Build Array (concatenate)(w523, w524) -> (w522:T6)
                }
              }
            }
            n351 = control-ref of="Карта 2"() -> (w506:refnum<vi>)
            n352 = property class="XYGraph (strict)"(reference=w506, "AnntList"=w490) -> ()  [unwired: 1 in, 2 out]
          }
        }
      }
      event "Перемешать соотношения": Value Change {
        n353 = event-data() -> ()  [unwired: 1 in, 3 out]
        n354 = case shown="True" "Перемешать соотношения" {
          frame False {
          }
          frame True {
            n355 = control-ref of="Все возможные точки карты"() -> (w870:refnum<vi>)
            n356 = property class="Arr (strict)"(reference=w870) -> (reference out=w866:refnum<vi>, "Value"=w867:cluster{"I":dbl, "Q":dbl, "ПБ":u32}[])  [unwired: 1 in, 1 out]
            n357 = for {
              tunnel: w867 -> [w894] mode=indexing
              tunnel: [w893] -> w869 mode=indexing
              n358 = Unbundle By Name(w894) -> ("ПБ"=w893:u32)
            }
            n359 = Array Size(array=w869) -> (size(s)=w863:i32)
            n360 = Decrement(x=w863) -> (x-1=w864:i32)
            n361 = for {
              N: w864 -> [_]
              shift-right: [w875] -> w868
              shift-left: w869 -> [w879]
              shift-right: [w873] -> _
              shift-left: w863 -> [w874]
              n362 = To Double Precision Float(number=w874) -> (double precision float=w871:dbl)
              n363 = Random Number (0-1)() -> (number: 0 to 1=w880:dbl)
              n364 = Multiply(x=w871, y=w880) -> (x*y=w878:dbl)
              n365 = Round Toward -Infinity(1:w878) -> (0:w877:dbl)
              n366 = To Long Integer(number=w877) -> (32bit integer=w872:i32)
              n367 = Decrement(x=w874) -> (x-1=w873:i32)
              n368 = Not Equal?(x=w873, y=w872) -> (x != y?=w876:bool)
              n369 = case shown="True" w876 {
                tunnel: w879 -> [w881 w885]
                tunnel: [w881 w884] -> w875
                tunnel: w873 -> [_ w883]
                tunnel: w872 -> [_ w882]
                frame False {
                }
                frame True {
                  n370 = in-place {
                    n371 = in-place-array #2(w885, w883, w882) -> (w889:u32, w888:u32)
                    n372 = Swap Values(12:w889, 14:w888) -> (1:w887:u32, 3:w886:u32)  [unwired: 1 in]
                    n373 = in-place-array #2(w887, w886) -> (w884:u32[])  [unwired: 2 out]
                  }
                }
              }
            }
            n374 = for {
              tunnel: w868 -> [w892] mode=indexing
              tunnel: [w891] -> w865 mode=indexing
              tunnel: w867 -> [w890] mode=indexing
              n375 = Bundle By Name(cluster=w890, "ПБ"=w892) -> (w891:cluster{"I":dbl, "Q":dbl, "ПБ":u32})
            }
            n376 = property class="Arr (strict)"(reference=w866, "Value"=w865) -> ()  [unwired: 1 in, 2 out]
          }
        }
      }
      event "Сохранить карту в файл": Value Change {
        n377 = event-data() -> ()  [unwired: 1 in, 1 out]
        n378 = case shown="True" "Сохранить карту в файл" {
          tunnel: w895 -> [_ w899]
          frame False {
          }
          frame True {
            n379 = control-ref of="Точки карты (позиции)"() -> (w906:refnum<vi>)
            n380 = control-ref of="Размер карты (N*N)"() -> (w908:refnum<vi>)
            n381 = property class="Slide (strict)"(reference=w908) -> ("Value"=w909:i32)  [unwired: 1 in, 2 out]
            n382 = property class="Arr (strict)"(reference=w906) -> ("Value"=w907:bool[][])  [unwired: 1 in, 2 out]
            n383 = for {
              N: w909 -> [w955]
              tunnel: w907 -> [w957] mode=indexing
              tunnel: [w956] -> w910 mode=indexing
              n384 = for {
                N: w955 -> [_]
                tunnel: w957 -> [w958] mode=indexing
                tunnel: [w959] -> w956 mode=indexing
                n385 = Boolean To (0,1)(Boolean=w958) -> (0, 1=w959:i16)
              }
            }
            n386 = control-ref of="Все возможные точки карты"() -> (w902:refnum<vi>)
            n387 = control-ref of="Соотношение точек с ПБ"() -> (w900:refnum<vi>)
            n388 = control-ref of="Интервалы и смещения"() -> (w904:refnum<vi>)
            n389 = property class="Clust (strict)"(reference=w904) -> ("Value"=w905:T1)  [unwired: 1 in, 2 out]
            n390 = property class="Ring (strict)"(reference=w900) -> ("Value"=w901:u8)  [unwired: 1 in, 2 out]
            n391 = property class="Arr (strict)"(reference=w902) -> ("Value"=w903:cluster{"I":dbl, "Q":dbl, "ПБ":u32}[])  [unwired: 1 in, 2 out]
            n392 = Bundle(cluster=w899, w910, "Value"=w905, "Value"=w903, "Value"=w901) -> (w913:T2)
            n393 = Flatten To XML(anything=w913) -> (xml string=w912:string)
            n394 = case shown="No Error" errorcluster {"status"=FALSE, "code"=0, "source"=""} ("error in (no error)") {
              selector: errorcluster {"status"=FALSE, "code"=0, "source"=""} ("error in (no error)") -> [w928 w954]
              tunnel: [w929 w954] -> w911
              tunnel: w912 -> [w940 w953]
              tunnel: [w927 w953] -> _
              tunnel: [w923 w952] -> w914
              tunnel: "Путь для сохранения карты" -> [w933 w952]
              tunnel: "" ("XML Encoding") -> [w945 _]
              frame No Error {
                n395 = Empty String/Path?(string/path=w945) -> (empty?=w944:bool)
                n396 = Concatenate Strings(" encoding='", w945, "' " ("Substring")) -> (w943:string)
                n397 = Select(t="", s=w944, f=w943) -> (s? t:f=w941:string)
                n398 = property class="App"() -> ("App.Version"=w938:string)  [unwired: 2 in, 2 out]
                n399 = Concatenate Strings("<?xml version='1.0' " ("XML Header"), w941, "standalone='yes' " ("Substring"), "?>" ("Substring"), "\r\n") -> (w949:string)
                n400 = Concatenate Strings("<Version>", w938, "</Version>", "\r\n") -> (w935:string)
                n401 = call <vilib>:"Open_Create_Replace File.vi"("advisory dialog? (display:T)"=FALSE, "pattern"="*.xml", "prompt"="Выберите путь к XML файлу карты" ("Prompt"), "error in (no error)"=w928, "function (open:0)"=T4."create or replace", "file path"=w933) -> ("error out"=w931:errorcluster, "refnum"=w926:refnum<file>)  [unwired: 2 in, 2 out]
                n402 = Concatenate Strings(w949, "<LVData xmlns=\"http://www.ni.com/LVData\">" ("Substring"), "\r\n", w935, w940, "</LVData>" ("Substring")) -> (w927:string)
                n403 = Write to Binary File(file (use dialog)=w926, data=w927, error in=w931, 5:FALSE ("prepend array or string size? (T)")) -> (refnum out=w924:refnum<file>, error out=w930:errorcluster)  [unwired: 3 out]
                n404 = Close File(refnum=w924, error in=w930) -> (path=w923:path, error out=w929:errorcluster)
              }
              frame Error {
              }
            }
            n405 = control-ref of="Путь для сохранения карты"() -> (w916:refnum<vi>)
            n406 = property class="Path"(reference=w916, "Value"=w914) -> ()  [unwired: 1 in, 2 out]
            n407 = case shown="No Error" w911 {
              selector: w911 -> [_ w962]
              frame No Error {
                n408 = One Button Dialog(message="Карта успешно сохранена.") -> ()  [unwired: 1 in, 1 out]
              }
              frame Error {
                n409 = call <vilib>:"General Error Handler.vi"("error in (no error)"=w962) -> ("error?"=w961:bool)  [unwired: 10 in, 4 out]
                n410 = Stop(stop? (T)=w961) -> ()
              }
            }
          }
        }
      }
      event "Заполнить полностью": Value Change {
        n411 = event-data() -> ()  [unwired: 1 in, 1 out]
        n412 = control-ref of="Размер карты (N*N)"() -> (w964:refnum<vi>)
        n413 = control-ref of="Точки карты (позиции)"() -> (w965:refnum<vi>)
        n414 = property class="Slide (strict)"(reference=w964) -> ("Value"=w963:i32)  [unwired: 1 in, 2 out]
        n415 = case shown="True" "Заполнить полностью" {
          tunnel: w965 -> [_ w968]
          tunnel: w963 -> [_ w967]
          frame False {
          }
          frame True {
            n416 = Initialize Array(TRUE, w967, w967) -> (w969:bool[][])
            n417 = property class="Arr (strict)"(reference=w968, "Value"=w969) -> ()  [unwired: 1 in, 2 out]
          }
        }
      }
      event "Очистить полностью": Value Change {
        n418 = event-data() -> ()  [unwired: 1 in, 1 out]
        n419 = control-ref of="Размер карты (N*N)"() -> (w972:refnum<vi>)
        n420 = control-ref of="Точки карты (позиции)"() -> (w973:refnum<vi>)
        n421 = property class="Slide (strict)"(reference=w972) -> ("Value"=w971:i32)  [unwired: 1 in, 2 out]
        n422 = case shown="True" "Очистить полностью" {
          tunnel: w973 -> [_ w976]
          tunnel: w971 -> [_ w975]
          frame False {
          }
          frame True {
            n423 = Initialize Array(FALSE, w975, w975) -> (w977:bool[][])
            n424 = property class="Arr (strict)"(reference=w976, "Value"=w977) -> ()  [unwired: 1 in, 2 out]
          }
        }
      }
      event Timeout {
        n425 = event-data() -> ()  [unwired: 1 in, 1 out]
      }
    }
  }
